vi "Downcast Object.vi"(8 "error in (no error)":errorcluster, 9 "Data Type":u8(ring)=2 items=["DTYPE_BU"=2, "DTYPE_WU"=3, "DTYPE_LU"=4, "DTYPE_QU"=5, "DTYPE_OU"=25, "DTYPE_B"=6, "DTYPE_W"=7, "DTYPE_L"=8, "DTYPE_Q"=9, "DTYPE_O"=26, "DTYPE_FLOAT"=52, "DTYPE_DOUBLE"=53, "DTYPE_T"=14, "DTYPE_IDENT"=191, "DTYPE_NID"=192, "DTYPE_PATH"=193, "DTYPE_PARAM"=194, "DTYPE_SIGNAL"=195, "DTYPE_DIMENSION"=196, "DTYPE_WINDOW"=197, "DTYPE_SLOPE"=198, "DTYPE_FUNCTION"=199, "DTYPE_CONGLOM"=200, "DTYPE_RANGE"=201, "DTYPE_ACTION"=202, "DTYPE_DISPATCH"=203, "DTYPE_PROGRAM"=204, "DTYPE_ROUTINE"=205, "DTYPE_PROCEDURE"=206, "DTYPE_METHOD"=207, "DTYPE_DEPENDENCY"=208, "DTYPE_CONDITION"=209, "DTYPE_EVENT"=210, "DTYPE_WITH_UNITS"=211, "DTYPE_CALL"=212, "DTYPE_WITH_ERROR"=213, "DTYPE_LIST"=214, "DTYPE_TUPLE"=215, "DTYPE_DICTIONARY"=216, "DTYPE_POINTER"=51, "DTYPE_DSC"=24], 10 "Class Type":u8(ring)=2 items=["CLASS_S"=1, "CLASS_D"=2, "CLASS_A"=4, "CLASS_R"=194, "CLASS_APD"=196], 11 "Data in":refnum<class "Data.lvclass">) -> (0 "error out":errorcluster, 3 "Data out":refnum<class "Data.lvclass">)   [LabVIEW 2013, in "MDSplus.lvlib" / "Data.lvclass"]
uses:
  <vilib>/MDSplus/Classes/Data_Class/Data.lvclass
  <vilib>/MDSplus/Classes/Data_Class/Scalar_Class/Float32_Class/Float32.lvclass
  <vilib>/MDSplus/Classes/Data_Class/Scalar_Class/Uint8_Class/Uint8.lvclass
  <vilib>/MDSplus/Classes/Data_Class/Scalar_Class/Uint16_Class/Uint16.lvclass
  <vilib>/MDSplus/Classes/Data_Class/Scalar_Class/Uint32_Class/Uint32.lvclass
  <vilib>/MDSplus/Classes/Data_Class/Scalar_Class/Uint64_Class/Uint64.lvclass
  <vilib>/MDSplus/Classes/Data_Class/Scalar_Class/Int8_Class/Int8.lvclass
  <vilib>/MDSplus/Classes/Data_Class/Scalar_Class/Int16_Class/Int16.lvclass
  <vilib>/MDSplus/Classes/Data_Class/Scalar_Class/Int32_Class/Int32.lvclass
  <vilib>/MDSplus/Classes/Data_Class/Scalar_Class/Int64_Class/Int64.lvclass
  <vilib>/MDSplus/Classes/Data_Class/Scalar_Class/String_Class/String.lvclass
  <vilib>/MDSplus/Classes/Data_Class/Scalar_Class/Float64_Class/Float64.lvclass
  <vilib>/MDSplus/Classes/Data_Class/Array_Class/Uint8Array_Class/Uint8Array.lvclass
  <vilib>/MDSplus/Classes/Data_Class/Array_Class/Uint16Array_Class/Uint16Array.lvclass
  <vilib>/MDSplus/Classes/Data_Class/Array_Class/Uint32Array_Class/Uint32Array.lvclass
  <vilib>/MDSplus/Classes/Data_Class/Array_Class/Uint64Array_Class/Uint64Array.lvclass
  <vilib>/MDSplus/Classes/Data_Class/Array_Class/Int8Array_Class/Int8Array.lvclass
  <vilib>/MDSplus/Classes/Data_Class/Array_Class/Int16Array_Class/Int16Array.lvclass
  <vilib>/MDSplus/Classes/Data_Class/Array_Class/Int32Array_Class/Int32Array.lvclass
  <vilib>/MDSplus/Classes/Data_Class/Array_Class/Int64Array_Class/Int64Array.lvclass
  <vilib>/MDSplus/Classes/Data_Class/Array_Class/StringArray_Class/StringArray.lvclass
  <vilib>/MDSplus/Classes/Data_Class/Array_Class/Float32Array_Class/Float32Array.lvclass
  <vilib>/MDSplus/Classes/Data_Class/Array_Class/Float64Array_Class/Float64Array.lvclass
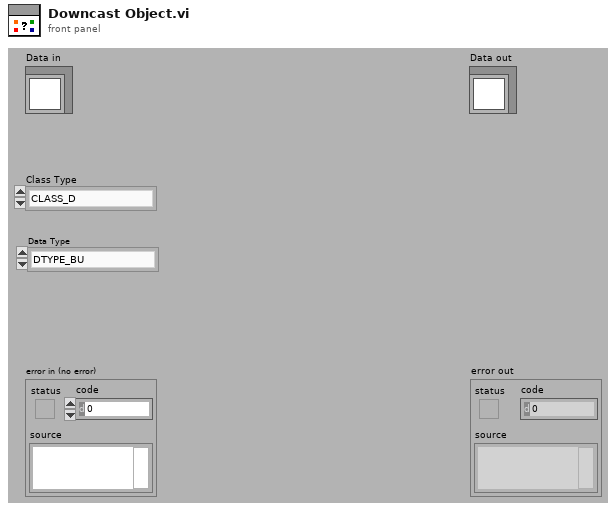
[diagram p1: front panel]
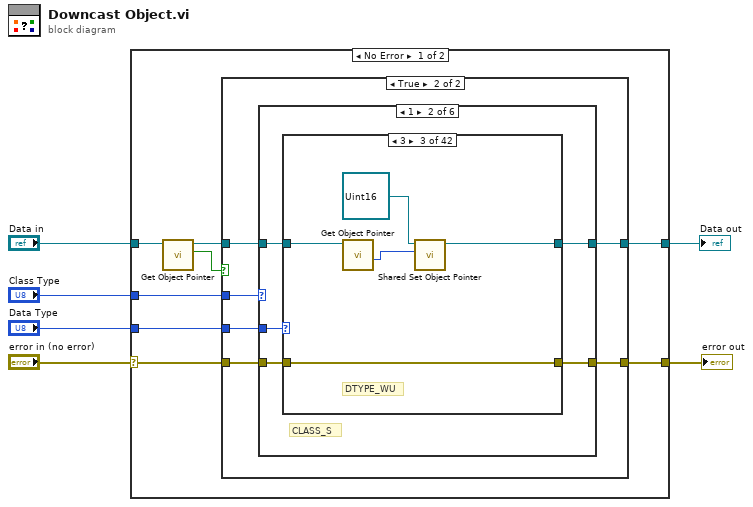
[diagram p0: block diagram]
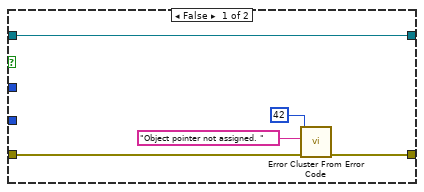
[diagram p2: hidden frame]
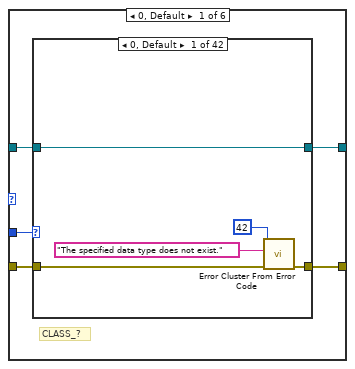
[diagram p3: hidden frame]
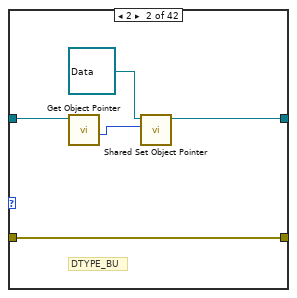
[diagram p4: hidden frame]
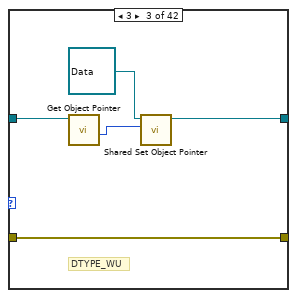
[diagram p5: hidden frame]
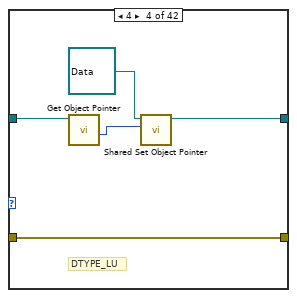
[diagram p6: hidden frame]
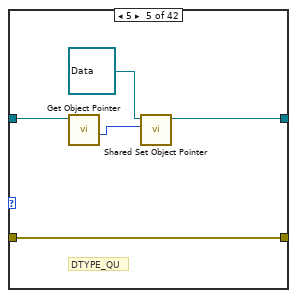
[diagram p7: hidden frame]
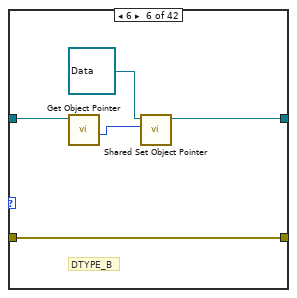
[diagram p8: hidden frame]
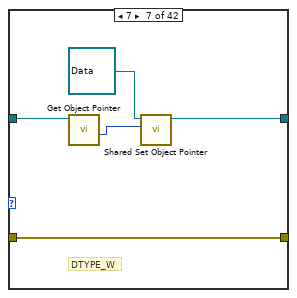
[diagram p9: hidden frame]
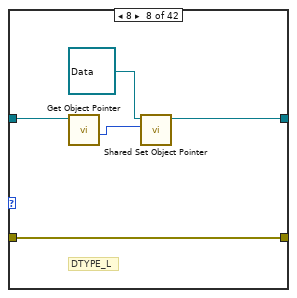
[diagram p10: hidden frame]
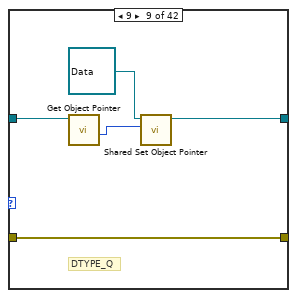
[diagram p11: hidden frame]
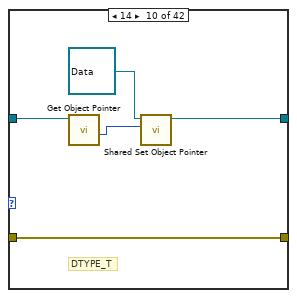
[diagram p12: hidden frame]
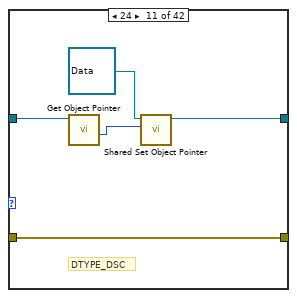
[diagram p13: hidden frame]
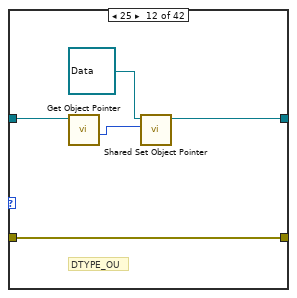
[diagram p14: hidden frame]
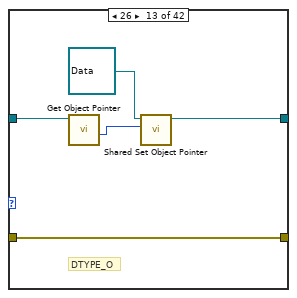
[diagram p15: hidden frame]
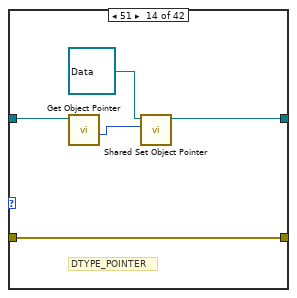
[diagram p16: hidden frame]
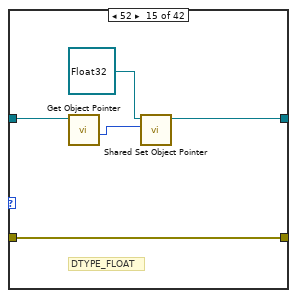
[diagram p17: hidden frame]
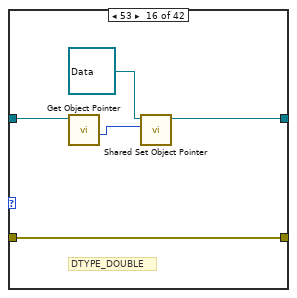
[diagram p18: hidden frame]
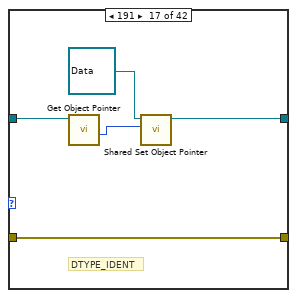
[diagram p19: hidden frame]
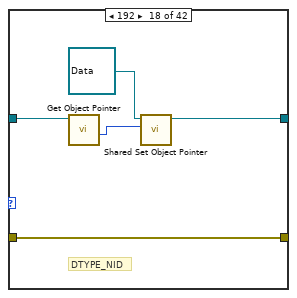
[diagram p20: hidden frame]
diagram:
  n1 = case shown="No Error" "error in (no error)" {
    selector: "error in (no error)" -> [w12 w1317]
    tunnel: [w11 w1317] -> w5
    tunnel: [w10 w1316] -> w3
    tunnel: "Data in" -> [w9 w1316]
    tunnel: "Class Type" -> [w13 _]
    tunnel: "Data Type" -> [w14 _]
    frame No Error {
      n2 = call-dynamic "Get Object Pointer.vi"("Data in"=w9) -> ("Assigned object pointer?"=w7:bool, "Data out"=w8:refnum<class "Data.lvclass">)  [unwired: 8 in, 1 out]
      n3 = case shown="True" w7 {
        tunnel: w14 -> [_ w25]
        tunnel: w13 -> [_ w24]
        tunnel: w12 -> [w17 w23]
        tunnel: [w16 w22] -> w11
        tunnel: [w15 w21] -> w10
        tunnel: w8 -> [w15 w20]
        frame False {
          n4 = call <vilib>:"Error Cluster From Error Code.vi"("error in (no error)"=w17, "error message (\"\")"="Object pointer not assigned. " ("error message (\"\")"), "error code (0)"=42) -> ("error out"=w16:errorcluster)  [unwired: 6 in]
        }
        frame True {
          n5 = case shown="1" w24 {
            tunnel: w20 -> [w27 w242 w457 w672 w887 w1102]
            tunnel: w25 -> [w30 w245 w460 w675 w890 w1105]
            tunnel: w23 -> [w29 w244 w459 w674 w889 w1104]
            tunnel: [w28 w243 w458 w673 w888 w1103] -> w22
            tunnel: [w26 w241 w456 w671 w886 w1101] -> w21
            frame 0, Default {
              # "CLASS_?"
              n6 = case shown="0, Default" w30 {
                tunnel: w29 -> [w35 w37 w42 w47 w52 w57 w62 w67 w72 w77 w82 w87 w92 w97 w102 w107 w112 w117 w122 w127 w132 w137 w142 w147 w152 w157 w162 w167 w172 w177 w182 w187 w192 w197 w202 w207 w212 w217 w222 w227 w232 w237]
                tunnel: [w33 w37 w42 w47 w52 w57 w62 w67 w72 w77 w82 w87 w92 w97 w102 w107 w112 w117 w122 w127 w132 w137 w142 w147 w152 w157 w162 w167 w172 w177 w182 w187 w192 w197 w202 w207 w212 w217 w222 w227 w232 w237] -> w28
                tunnel: [w32 w38 w43 w48 w53 w58 w63 w68 w73 w78 w83 w88 w93 w98 w104 w109 w114 w119 w124 w129 w134 w139 w144 w149 w154 w159 w164 w169 w174 w179 w184 w189 w194 w199 w204 w209 w214 w219 w224 w229 w234 w239] -> w26
                tunnel: w27 -> [w32 w40 w44 w49 w54 w59 w64 w69 w74 w79 w84 w89 w94 w99 w105 w110 w115 w120 w125 w130 w135 w140 w145 w150 w155 w160 w165 w170 w175 w180 w185 w190 w195 w200 w205 w210 w215 w220 w225 w230 w235 w240]
                frame 0, Default {
                  n7 = call <vilib>:"Error Cluster From Error Code.vi"("error in (no error)"=w35, "error message (\"\")"="The specified data type does not exist." ("error message (\"\")"), "error code (0)"=42) -> ("error out"=w33:errorcluster)  [unwired: 6 in]
                }
                frame 2 {
                  # "DTYPE_BU"
                  n8 = call-dynamic "Get Object Pointer.vi"("Data in"=w40) -> ("Object Pointer"=w36:i64)  [unwired: 8 in, 2 out]
                  n9 = call <vilib>:"Shared Set Object Pointer.vi"("Object Pointer"=w36, "Data in"=refnum<class "Data.lvclass"> refnum ("Data.lvclass")) -> ("Data out"=w38:refnum<class "Data.lvclass">)  [unwired: 9 in]
                }
                frame 3 {
                  # "DTYPE_WU"
                  n10 = call-dynamic "Get Object Pointer.vi"("Data in"=w44) -> ("Object Pointer"=w41:i64)  [unwired: 8 in, 2 out]
                  n11 = call <vilib>:"Shared Set Object Pointer.vi"("Object Pointer"=w41, "Data in"=refnum<class "Data.lvclass"> refnum ("Data.lvclass")) -> ("Data out"=w43:refnum<class "Data.lvclass">)  [unwired: 9 in]
                }
                frame 4 {
                  # "DTYPE_LU"
                  n12 = call-dynamic "Get Object Pointer.vi"("Data in"=w49) -> ("Object Pointer"=w46:i64)  [unwired: 8 in, 2 out]
                  n13 = call <vilib>:"Shared Set Object Pointer.vi"("Object Pointer"=w46, "Data in"=refnum<class "Data.lvclass"> refnum ("Data.lvclass")) -> ("Data out"=w48:refnum<class "Data.lvclass">)  [unwired: 9 in]
                }
                frame 5 {
                  # "DTYPE_QU"
                  n14 = call-dynamic "Get Object Pointer.vi"("Data in"=w54) -> ("Object Pointer"=w51:i64)  [unwired: 8 in, 2 out]
                  n15 = call <vilib>:"Shared Set Object Pointer.vi"("Object Pointer"=w51, "Data in"=refnum<class "Data.lvclass"> refnum ("Data.lvclass")) -> ("Data out"=w53:refnum<class "Data.lvclass">)  [unwired: 9 in]
                }
                frame 6 {
                  # "DTYPE_B"
                  n16 = call-dynamic "Get Object Pointer.vi"("Data in"=w59) -> ("Object Pointer"=w56:i64)  [unwired: 8 in, 2 out]
                  n17 = call <vilib>:"Shared Set Object Pointer.vi"("Object Pointer"=w56, "Data in"=refnum<class "Data.lvclass"> refnum ("Data.lvclass")) -> ("Data out"=w58:refnum<class "Data.lvclass">)  [unwired: 9 in]
                }
                frame 7 {
                  # "DTYPE_W"
                  n18 = call-dynamic "Get Object Pointer.vi"("Data in"=w64) -> ("Object Pointer"=w61:i64)  [unwired: 8 in, 2 out]
                  n19 = call <vilib>:"Shared Set Object Pointer.vi"("Object Pointer"=w61, "Data in"=refnum<class "Data.lvclass"> refnum ("Data.lvclass")) -> ("Data out"=w63:refnum<class "Data.lvclass">)  [unwired: 9 in]
                }
                frame 8 {
                  # "DTYPE_L"
                  n20 = call-dynamic "Get Object Pointer.vi"("Data in"=w69) -> ("Object Pointer"=w66:i64)  [unwired: 8 in, 2 out]
                  n21 = call <vilib>:"Shared Set Object Pointer.vi"("Object Pointer"=w66, "Data in"=refnum<class "Data.lvclass"> refnum ("Data.lvclass")) -> ("Data out"=w68:refnum<class "Data.lvclass">)  [unwired: 9 in]
                }
                frame 9 {
                  # "DTYPE_Q"
                  n22 = call-dynamic "Get Object Pointer.vi"("Data in"=w74) -> ("Object Pointer"=w71:i64)  [unwired: 8 in, 2 out]
                  n23 = call <vilib>:"Shared Set Object Pointer.vi"("Object Pointer"=w71, "Data in"=refnum<class "Data.lvclass"> refnum ("Data.lvclass")) -> ("Data out"=w73:refnum<class "Data.lvclass">)  [unwired: 9 in]
                }
                frame 14 {
                  # "DTYPE_T"
                  n24 = call-dynamic "Get Object Pointer.vi"("Data in"=w79) -> ("Object Pointer"=w76:i64)  [unwired: 8 in, 2 out]
                  n25 = call <vilib>:"Shared Set Object Pointer.vi"("Object Pointer"=w76, "Data in"=refnum<class "Data.lvclass"> refnum ("Data.lvclass")) -> ("Data out"=w78:refnum<class "Data.lvclass">)  [unwired: 9 in]
                }
                frame 24 {
                  # "DTYPE_DSC"
                  n26 = call-dynamic "Get Object Pointer.vi"("Data in"=w84) -> ("Object Pointer"=w81:i64)  [unwired: 8 in, 2 out]
                  n27 = call <vilib>:"Shared Set Object Pointer.vi"("Object Pointer"=w81, "Data in"=refnum<class "Data.lvclass"> refnum ("Data.lvclass")) -> ("Data out"=w83:refnum<class "Data.lvclass">)  [unwired: 9 in]
                }
                frame 25 {
                  # "DTYPE_OU"
                  n28 = call-dynamic "Get Object Pointer.vi"("Data in"=w89) -> ("Object Pointer"=w86:i64)  [unwired: 8 in, 2 out]
                  n29 = call <vilib>:"Shared Set Object Pointer.vi"("Object Pointer"=w86, "Data in"=refnum<class "Data.lvclass"> refnum ("Data.lvclass")) -> ("Data out"=w88:refnum<class "Data.lvclass">)  [unwired: 9 in]
                }
                frame 26 {
                  # "DTYPE_O"
                  n30 = call-dynamic "Get Object Pointer.vi"("Data in"=w94) -> ("Object Pointer"=w91:i64)  [unwired: 8 in, 2 out]
                  n31 = call <vilib>:"Shared Set Object Pointer.vi"("Object Pointer"=w91, "Data in"=refnum<class "Data.lvclass"> refnum ("Data.lvclass")) -> ("Data out"=w93:refnum<class "Data.lvclass">)  [unwired: 9 in]
                }
                frame 51 {
                  # "DTYPE_POINTER"
                  n32 = call-dynamic "Get Object Pointer.vi"("Data in"=w99) -> ("Object Pointer"=w96:i64)  [unwired: 8 in, 2 out]
                  n33 = call <vilib>:"Shared Set Object Pointer.vi"("Object Pointer"=w96, "Data in"=refnum<class "Data.lvclass"> refnum ("Data.lvclass")) -> ("Data out"=w98:refnum<class "Data.lvclass">)  [unwired: 9 in]
                }
                frame 52 {
                  # "DTYPE_FLOAT"
                  n34 = call-dynamic "Get Object Pointer.vi"("Data in"=w105) -> ("Object Pointer"=w101:i64)  [unwired: 8 in, 2 out]
                  n35 = call <vilib>:"Shared Set Object Pointer.vi"("Object Pointer"=w101, "Data in"=refnum<class "Float32.lvclass"> refnum ("Float32.lvclass")) -> ("Data out"=w104:refnum<class "Float32.lvclass">)  [unwired: 9 in]
                }
                frame 53 {
                  # "DTYPE_DOUBLE"
                  n36 = call-dynamic "Get Object Pointer.vi"("Data in"=w110) -> ("Object Pointer"=w106:i64)  [unwired: 8 in, 2 out]
                  n37 = call <vilib>:"Shared Set Object Pointer.vi"("Object Pointer"=w106, "Data in"=refnum<class "Data.lvclass"> refnum ("Data.lvclass")) -> ("Data out"=w109:refnum<class "Data.lvclass">)  [unwired: 9 in]
                }
                frame 191 {
                  # "DTYPE_IDENT"
                  n38 = call-dynamic "Get Object Pointer.vi"("Data in"=w115) -> ("Object Pointer"=w111:i64)  [unwired: 8 in, 2 out]
                  n39 = call <vilib>:"Shared Set Object Pointer.vi"("Object Pointer"=w111, "Data in"=refnum<class "Data.lvclass"> refnum ("Data.lvclass")) -> ("Data out"=w114:refnum<class "Data.lvclass">)  [unwired: 9 in]
                }
                frame 192 {
                  # "DTYPE_NID"
                  n40 = call-dynamic "Get Object Pointer.vi"("Data in"=w120) -> ("Object Pointer"=w116:i64)  [unwired: 8 in, 2 out]
                  n41 = call <vilib>:"Shared Set Object Pointer.vi"("Object Pointer"=w116, "Data in"=refnum<class "Data.lvclass"> refnum ("Data.lvclass")) -> ("Data out"=w119:refnum<class "Data.lvclass">)  [unwired: 9 in]
                }
                frame 193 {
                  # "DTYPE_PATH"
                  n42 = call-dynamic "Get Object Pointer.vi"("Data in"=w125) -> ("Object Pointer"=w121:i64)  [unwired: 8 in, 2 out]
                  n43 = call <vilib>:"Shared Set Object Pointer.vi"("Object Pointer"=w121, "Data in"=refnum<class "Data.lvclass"> refnum ("Data.lvclass")) -> ("Data out"=w124:refnum<class "Data.lvclass">)  [unwired: 9 in]
                }
                frame 194 {
                  # "DTYPE_PARAM"
                  n44 = call-dynamic "Get Object Pointer.vi"("Data in"=w130) -> ("Object Pointer"=w126:i64)  [unwired: 8 in, 2 out]
                  n45 = call <vilib>:"Shared Set Object Pointer.vi"("Object Pointer"=w126, "Data in"=refnum<class "Data.lvclass"> refnum ("Data.lvclass")) -> ("Data out"=w129:refnum<class "Data.lvclass">)  [unwired: 9 in]
                }
                frame 195 {
                  # "DTYPE_SIGNAL"
                  n46 = call-dynamic "Get Object Pointer.vi"("Data in"=w135) -> ("Object Pointer"=w131:i64)  [unwired: 8 in, 2 out]
                  n47 = call <vilib>:"Shared Set Object Pointer.vi"("Object Pointer"=w131, "Data in"=refnum<class "Data.lvclass"> refnum ("Data.lvclass")) -> ("Data out"=w134:refnum<class "Data.lvclass">)  [unwired: 9 in]
                }
                frame 196 {
                  # "DTYPE_DIMENSION"
                  n48 = call-dynamic "Get Object Pointer.vi"("Data in"=w140) -> ("Object Pointer"=w136:i64)  [unwired: 8 in, 2 out]
                  n49 = call <vilib>:"Shared Set Object Pointer.vi"("Object Pointer"=w136, "Data in"=refnum<class "Data.lvclass"> refnum ("Data.lvclass")) -> ("Data out"=w139:refnum<class "Data.lvclass">)  [unwired: 9 in]
                }
                frame 197 {
                  # "DTYPE_WINDOW"
                  n50 = call-dynamic "Get Object Pointer.vi"("Data in"=w145) -> ("Object Pointer"=w141:i64)  [unwired: 8 in, 2 out]
                  n51 = call <vilib>:"Shared Set Object Pointer.vi"("Object Pointer"=w141, "Data in"=refnum<class "Data.lvclass"> refnum ("Data.lvclass")) -> ("Data out"=w144:refnum<class "Data.lvclass">)  [unwired: 9 in]
                }
                frame 198 {
                  # "DTYPE_SLOPE"
                  n52 = call-dynamic "Get Object Pointer.vi"("Data in"=w150) -> ("Object Pointer"=w146:i64)  [unwired: 8 in, 2 out]
                  n53 = call <vilib>:"Shared Set Object Pointer.vi"("Object Pointer"=w146, "Data in"=refnum<class "Data.lvclass"> refnum ("Data.lvclass")) -> ("Data out"=w149:refnum<class "Data.lvclass">)  [unwired: 9 in]
                }
                frame 199 {
                  # "DTYPE_FUNCTION"
                  n54 = call-dynamic "Get Object Pointer.vi"("Data in"=w155) -> ("Object Pointer"=w151:i64)  [unwired: 8 in, 2 out]
                  n55 = call <vilib>:"Shared Set Object Pointer.vi"("Object Pointer"=w151, "Data in"=refnum<class "Data.lvclass"> refnum ("Data.lvclass")) -> ("Data out"=w154:refnum<class "Data.lvclass">)  [unwired: 9 in]
                }
                frame 200 {
                  # "DTYPE_CONGLOM"
                  n56 = call-dynamic "Get Object Pointer.vi"("Data in"=w160) -> ("Object Pointer"=w156:i64)  [unwired: 8 in, 2 out]
                  n57 = call <vilib>:"Shared Set Object Pointer.vi"("Object Pointer"=w156, "Data in"=refnum<class "Data.lvclass"> refnum ("Data.lvclass")) -> ("Data out"=w159:refnum<class "Data.lvclass">)  [unwired: 9 in]
                }
                frame 201 {
                  # "DTYPE_RANGE"
                  n58 = call-dynamic "Get Object Pointer.vi"("Data in"=w165) -> ("Object Pointer"=w161:i64)  [unwired: 8 in, 2 out]
                  n59 = call <vilib>:"Shared Set Object Pointer.vi"("Object Pointer"=w161, "Data in"=refnum<class "Data.lvclass"> refnum ("Data.lvclass")) -> ("Data out"=w164:refnum<class "Data.lvclass">)  [unwired: 9 in]
                }
                frame 202 {
                  # "DTYPE_ACTION"
                  n60 = call-dynamic "Get Object Pointer.vi"("Data in"=w170) -> ("Object Pointer"=w166:i64)  [unwired: 8 in, 2 out]
                  n61 = call <vilib>:"Shared Set Object Pointer.vi"("Object Pointer"=w166, "Data in"=refnum<class "Data.lvclass"> refnum ("Data.lvclass")) -> ("Data out"=w169:refnum<class "Data.lvclass">)  [unwired: 9 in]
                }
                frame 203 {
                  # "DTYPE_DISPATCH"
                  n62 = call-dynamic "Get Object Pointer.vi"("Data in"=w175) -> ("Object Pointer"=w171:i64)  [unwired: 8 in, 2 out]
                  n63 = call <vilib>:"Shared Set Object Pointer.vi"("Object Pointer"=w171, "Data in"=refnum<class "Data.lvclass"> refnum ("Data.lvclass")) -> ("Data out"=w174:refnum<class "Data.lvclass">)  [unwired: 9 in]
                }
                frame 204 {
                  # "DTYPE_PROGRAM"
                  n64 = call-dynamic "Get Object Pointer.vi"("Data in"=w180) -> ("Object Pointer"=w176:i64)  [unwired: 8 in, 2 out]
                  n65 = call <vilib>:"Shared Set Object Pointer.vi"("Object Pointer"=w176, "Data in"=refnum<class "Data.lvclass"> refnum ("Data.lvclass")) -> ("Data out"=w179:refnum<class "Data.lvclass">)  [unwired: 9 in]
                }
                frame 205 {
                  # "DTYPE_ROUTINE"
                  n66 = call-dynamic "Get Object Pointer.vi"("Data in"=w185) -> ("Object Pointer"=w181:i64)  [unwired: 8 in, 2 out]
                  n67 = call <vilib>:"Shared Set Object Pointer.vi"("Object Pointer"=w181, "Data in"=refnum<class "Data.lvclass"> refnum ("Data.lvclass")) -> ("Data out"=w184:refnum<class "Data.lvclass">)  [unwired: 9 in]
                }
                frame 206 {
                  # "DTYPE_PROCEDURE"
                  n68 = call-dynamic "Get Object Pointer.vi"("Data in"=w190) -> ("Object Pointer"=w186:i64)  [unwired: 8 in, 2 out]
                  n69 = call <vilib>:"Shared Set Object Pointer.vi"("Object Pointer"=w186, "Data in"=refnum<class "Data.lvclass"> refnum ("Data.lvclass")) -> ("Data out"=w189:refnum<class "Data.lvclass">)  [unwired: 9 in]
                }
                frame 207 {
                  # "DTYPE_METHOD"
                  n70 = call-dynamic "Get Object Pointer.vi"("Data in"=w195) -> ("Object Pointer"=w191:i64)  [unwired: 8 in, 2 out]
                  n71 = call <vilib>:"Shared Set Object Pointer.vi"("Object Pointer"=w191, "Data in"=refnum<class "Data.lvclass"> refnum ("Data.lvclass")) -> ("Data out"=w194:refnum<class "Data.lvclass">)  [unwired: 9 in]
                }
                frame 208 {
                  # "DTYPE_DEPENDENCY"
                  n72 = call-dynamic "Get Object Pointer.vi"("Data in"=w200) -> ("Object Pointer"=w196:i64)  [unwired: 8 in, 2 out]
                  n73 = call <vilib>:"Shared Set Object Pointer.vi"("Object Pointer"=w196, "Data in"=refnum<class "Data.lvclass"> refnum ("Data.lvclass")) -> ("Data out"=w199:refnum<class "Data.lvclass">)  [unwired: 9 in]
                }
                frame 209 {
                  # "DTYPE_CONDITION"
                  n74 = call-dynamic "Get Object Pointer.vi"("Data in"=w205) -> ("Object Pointer"=w201:i64)  [unwired: 8 in, 2 out]
                  n75 = call <vilib>:"Shared Set Object Pointer.vi"("Object Pointer"=w201, "Data in"=refnum<class "Data.lvclass"> refnum ("Data.lvclass")) -> ("Data out"=w204:refnum<class "Data.lvclass">)  [unwired: 9 in]
                }
                frame 210 {
                  # "DTYPE_EVENT"
                  n76 = call-dynamic "Get Object Pointer.vi"("Data in"=w210) -> ("Object Pointer"=w206:i64)  [unwired: 8 in, 2 out]
                  n77 = call <vilib>:"Shared Set Object Pointer.vi"("Object Pointer"=w206, "Data in"=refnum<class "Data.lvclass"> refnum ("Data.lvclass")) -> ("Data out"=w209:refnum<class "Data.lvclass">)  [unwired: 9 in]
                }
                frame 211 {
                  # "DTYPE_WITH_UNITS"
                  n78 = call-dynamic "Get Object Pointer.vi"("Data in"=w215) -> ("Object Pointer"=w211:i64)  [unwired: 8 in, 2 out]
                  n79 = call <vilib>:"Shared Set Object Pointer.vi"("Object Pointer"=w211, "Data in"=refnum<class "Data.lvclass"> refnum ("Data.lvclass")) -> ("Data out"=w214:refnum<class "Data.lvclass">)  [unwired: 9 in]
                }
                frame 212 {
                  # "DTYPE_CALL"
                  n80 = call-dynamic "Get Object Pointer.vi"("Data in"=w220) -> ("Object Pointer"=w216:i64)  [unwired: 8 in, 2 out]
                  n81 = call <vilib>:"Shared Set Object Pointer.vi"("Object Pointer"=w216, "Data in"=refnum<class "Data.lvclass"> refnum ("Data.lvclass")) -> ("Data out"=w219:refnum<class "Data.lvclass">)  [unwired: 9 in]
                }
                frame 213 {
                  # "DTYPE_WITH_ERROR"
                  n82 = call-dynamic "Get Object Pointer.vi"("Data in"=w225) -> ("Object Pointer"=w221:i64)  [unwired: 8 in, 2 out]
                  n83 = call <vilib>:"Shared Set Object Pointer.vi"("Object Pointer"=w221, "Data in"=refnum<class "Data.lvclass"> refnum ("Data.lvclass")) -> ("Data out"=w224:refnum<class "Data.lvclass">)  [unwired: 9 in]
                }
                frame 214 {
                  # "DTYPE_LIST"
                  n84 = call-dynamic "Get Object Pointer.vi"("Data in"=w230) -> ("Object Pointer"=w226:i64)  [unwired: 8 in, 2 out]
                  n85 = call <vilib>:"Shared Set Object Pointer.vi"("Object Pointer"=w226, "Data in"=refnum<class "Data.lvclass"> refnum ("Data.lvclass")) -> ("Data out"=w229:refnum<class "Data.lvclass">)  [unwired: 9 in]
                }
                frame 215 {
                  # "DTYPE_TUPLE"
                  n86 = call-dynamic "Get Object Pointer.vi"("Data in"=w235) -> ("Object Pointer"=w231:i64)  [unwired: 8 in, 2 out]
                  n87 = call <vilib>:"Shared Set Object Pointer.vi"("Object Pointer"=w231, "Data in"=refnum<class "Data.lvclass"> refnum ("Data.lvclass")) -> ("Data out"=w234:refnum<class "Data.lvclass">)  [unwired: 9 in]
                }
                frame 216 {
                  # "DTYPE_DICTIONARY"
                  n88 = call-dynamic "Get Object Pointer.vi"("Data in"=w240) -> ("Object Pointer"=w236:i64)  [unwired: 8 in, 2 out]
                  n89 = call <vilib>:"Shared Set Object Pointer.vi"("Object Pointer"=w236, "Data in"=refnum<class "Data.lvclass"> refnum ("Data.lvclass")) -> ("Data out"=w239:refnum<class "Data.lvclass">)  [unwired: 9 in]
                }
              }
            }
            frame 1 {
              # "CLASS_S"
              n90 = case shown="3" w245 {
                tunnel: w244 -> [w250 w252 w257 w262 w267 w272 w277 w282 w287 w292 w297 w302 w307 w312 w317 w322 w327 w332 w337 w342 w347 w352 w357 w362 w367 w372 w377 w382 w387 w392 w397 w402 w407 w412 w417 w422 w427 w432 w437 w442 w447 w452]
                tunnel: [w248 w252 w257 w262 w267 w272 w277 w282 w287 w292 w297 w302 w307 w312 w317 w322 w327 w332 w337 w342 w347 w352 w357 w362 w367 w372 w377 w382 w387 w392 w397 w402 w407 w412 w417 w422 w427 w432 w437 w442 w447 w452] -> w243
                tunnel: [w247 w253 w258 w263 w268 w273 w278 w283 w288 w293 w298 w303 w308 w313 w319 w324 w329 w334 w339 w344 w349 w354 w359 w364 w369 w374 w379 w384 w389 w394 w399 w404 w409 w414 w419 w424 w429 w434 w439 w444 w449 w454] -> w241
                tunnel: w242 -> [w247 w255 w259 w264 w269 w274 w279 w284 w289 w294 w299 w304 w309 w314 w320 w325 w330 w335 w340 w345 w350 w355 w360 w365 w370 w375 w380 w385 w390 w395 w400 w405 w410 w415 w420 w425 w430 w435 w440 w445 w450 w455]
                frame 0, Default {
                  n91 = call <vilib>:"Error Cluster From Error Code.vi"("error in (no error)"=w250, "error message (\"\")"="The specified data type does not exist." ("error message (\"\")"), "error code (0)"=42) -> ("error out"=w248:errorcluster)  [unwired: 6 in]
                }
                frame 2 {
                  # "DTYPE_BU"
                  n92 = call-dynamic "Get Object Pointer.vi"("Data in"=w255) -> ("Object Pointer"=w251:i64)  [unwired: 8 in, 2 out]
                  n93 = call <vilib>:"Shared Set Object Pointer.vi"("Object Pointer"=w251, "Data in"=refnum<class "Uint8.lvclass"> refnum ("Data.lvclass")) -> ("Data out"=w253:refnum<class "Uint8.lvclass">)  [unwired: 9 in]
                }
                frame 3 {
                  # "DTYPE_WU"
                  n94 = call-dynamic "Get Object Pointer.vi"("Data in"=w259) -> ("Object Pointer"=w256:i64)  [unwired: 8 in, 2 out]
                  n95 = call <vilib>:"Shared Set Object Pointer.vi"("Object Pointer"=w256, "Data in"=refnum<class "Uint16.lvclass"> refnum ("Data.lvclass")) -> ("Data out"=w258:refnum<class "Uint16.lvclass">)  [unwired: 9 in]
                }
                frame 4 {
                  # "DTYPE_LU"
                  n96 = call-dynamic "Get Object Pointer.vi"("Data in"=w264) -> ("Object Pointer"=w261:i64)  [unwired: 8 in, 2 out]
                  n97 = call <vilib>:"Shared Set Object Pointer.vi"("Object Pointer"=w261, "Data in"=refnum<class "Uint32.lvclass"> refnum ("Data.lvclass")) -> ("Data out"=w263:refnum<class "Uint32.lvclass">)  [unwired: 9 in]
                }
                frame 5 {
                  # "DTYPE_QU"
                  n98 = call-dynamic "Get Object Pointer.vi"("Data in"=w269) -> ("Object Pointer"=w266:i64)  [unwired: 8 in, 2 out]
                  n99 = call <vilib>:"Shared Set Object Pointer.vi"("Object Pointer"=w266, "Data in"=refnum<class "Uint64.lvclass"> refnum ("Data.lvclass")) -> ("Data out"=w268:refnum<class "Uint64.lvclass">)  [unwired: 9 in]
                }
                frame 6 {
                  # "DTYPE_B"
                  n100 = call-dynamic "Get Object Pointer.vi"("Data in"=w274) -> ("Object Pointer"=w271:i64)  [unwired: 8 in, 2 out]
                  n101 = call <vilib>:"Shared Set Object Pointer.vi"("Object Pointer"=w271, "Data in"=refnum<class "Int8.lvclass"> refnum ("Data.lvclass")) -> ("Data out"=w273:refnum<class "Int8.lvclass">)  [unwired: 9 in]
                }
                frame 7 {
                  # "DTYPE_W"
                  n102 = call-dynamic "Get Object Pointer.vi"("Data in"=w279) -> ("Object Pointer"=w276:i64)  [unwired: 8 in, 2 out]
                  n103 = call <vilib>:"Shared Set Object Pointer.vi"("Object Pointer"=w276, "Data in"=refnum<class "Int16.lvclass"> refnum ("Data.lvclass")) -> ("Data out"=w278:refnum<class "Int16.lvclass">)  [unwired: 9 in]
                }
                frame 8 {
                  # "DTYPE_L"
                  n104 = call-dynamic "Get Object Pointer.vi"("Data in"=w284) -> ("Object Pointer"=w281:i64)  [unwired: 8 in, 2 out]
                  n105 = call <vilib>:"Shared Set Object Pointer.vi"("Object Pointer"=w281, "Data in"=refnum<class "Int32.lvclass"> refnum ("Data.lvclass")) -> ("Data out"=w283:refnum<class "Int32.lvclass">)  [unwired: 9 in]
                }
                frame 9 {
                  # "DTYPE_Q"
                  n106 = call-dynamic "Get Object Pointer.vi"("Data in"=w289) -> ("Object Pointer"=w286:i64)  [unwired: 8 in, 2 out]
                  n107 = call <vilib>:"Shared Set Object Pointer.vi"("Object Pointer"=w286, "Data in"=refnum<class "Int64.lvclass"> refnum ("Data.lvclass")) -> ("Data out"=w288:refnum<class "Int64.lvclass">)  [unwired: 9 in]
                }
                frame 14 {
                  # "DTYPE_T"
                  n108 = call-dynamic "Get Object Pointer.vi"("Data in"=w294) -> ("Object Pointer"=w291:i64)  [unwired: 8 in, 2 out]
                  n109 = call <vilib>:"Shared Set Object Pointer.vi"("Object Pointer"=w291, "Data in"=refnum<class "String.lvclass"> refnum ("Data.lvclass")) -> ("Data out"=w293:refnum<class "String.lvclass">)  [unwired: 9 in]
                }
                frame 24 {
                  # "DTYPE_DSC"
                  n110 = call-dynamic "Get Object Pointer.vi"("Data in"=w299) -> ("Object Pointer"=w296:i64)  [unwired: 8 in, 2 out]
                  n111 = call <vilib>:"Shared Set Object Pointer.vi"("Object Pointer"=w296, "Data in"=refnum<class "Data.lvclass"> refnum ("Data.lvclass")) -> ("Data out"=w298:refnum<class "Data.lvclass">)  [unwired: 9 in]
                }
                frame 25 {
                  # "DTYPE_OU"
                  n112 = call-dynamic "Get Object Pointer.vi"("Data in"=w304) -> ("Object Pointer"=w301:i64)  [unwired: 8 in, 2 out]
                  n113 = call <vilib>:"Shared Set Object Pointer.vi"("Object Pointer"=w301, "Data in"=refnum<class "Data.lvclass"> refnum ("Data.lvclass")) -> ("Data out"=w303:refnum<class "Data.lvclass">)  [unwired: 9 in]
                }
                frame 26 {
                  # "DTYPE_O"
                  n114 = call-dynamic "Get Object Pointer.vi"("Data in"=w309) -> ("Object Pointer"=w306:i64)  [unwired: 8 in, 2 out]
                  n115 = call <vilib>:"Shared Set Object Pointer.vi"("Object Pointer"=w306, "Data in"=refnum<class "Data.lvclass"> refnum ("Data.lvclass")) -> ("Data out"=w308:refnum<class "Data.lvclass">)  [unwired: 9 in]
                }
                frame 51 {
                  # "DTYPE_POINTER"
                  n116 = call-dynamic "Get Object Pointer.vi"("Data in"=w314) -> ("Object Pointer"=w311:i64)  [unwired: 8 in, 2 out]
                  n117 = call <vilib>:"Shared Set Object Pointer.vi"("Object Pointer"=w311, "Data in"=refnum<class "Data.lvclass"> refnum ("Data.lvclass")) -> ("Data out"=w313:refnum<class "Data.lvclass">)  [unwired: 9 in]
                }
                frame 52 {
                  # "DTYPE_FLOAT"
                  n118 = call-dynamic "Get Object Pointer.vi"("Data in"=w320) -> ("Object Pointer"=w316:i64)  [unwired: 8 in, 2 out]
                  n119 = call <vilib>:"Shared Set Object Pointer.vi"("Object Pointer"=w316, "Data in"=refnum<class "Float32.lvclass"> refnum ("Float32.lvclass")) -> ("Data out"=w319:refnum<class "Float32.lvclass">)  [unwired: 9 in]
                }
                frame 53 {
                  # "DTYPE_DOUBLE"
                  n120 = call-dynamic "Get Object Pointer.vi"("Data in"=w325) -> ("Object Pointer"=w321:i64)  [unwired: 8 in, 2 out]
                  n121 = call <vilib>:"Shared Set Object Pointer.vi"("Object Pointer"=w321, "Data in"=refnum<class "Float64.lvclass"> refnum ("Data.lvclass")) -> ("Data out"=w324:refnum<class "Float64.lvclass">)  [unwired: 9 in]
                }
                frame 191 {
                  # "DTYPE_IDENT"
                  n122 = call-dynamic "Get Object Pointer.vi"("Data in"=w330) -> ("Object Pointer"=w326:i64)  [unwired: 8 in, 2 out]
                  n123 = call <vilib>:"Shared Set Object Pointer.vi"("Object Pointer"=w326, "Data in"=refnum<class "Data.lvclass"> refnum ("Data.lvclass")) -> ("Data out"=w329:refnum<class "Data.lvclass">)  [unwired: 9 in]
                }
                frame 192 {
                  # "DTYPE_NID"
                  n124 = call-dynamic "Get Object Pointer.vi"("Data in"=w335) -> ("Object Pointer"=w331:i64)  [unwired: 8 in, 2 out]
                  n125 = call <vilib>:"Shared Set Object Pointer.vi"("Object Pointer"=w331, "Data in"=refnum<class "Data.lvclass"> refnum ("Data.lvclass")) -> ("Data out"=w334:refnum<class "Data.lvclass">)  [unwired: 9 in]
                }
                frame 193 {
                  # "DTYPE_PATH"
                  n126 = call-dynamic "Get Object Pointer.vi"("Data in"=w340) -> ("Object Pointer"=w336:i64)  [unwired: 8 in, 2 out]
                  n127 = call <vilib>:"Shared Set Object Pointer.vi"("Object Pointer"=w336, "Data in"=refnum<class "Data.lvclass"> refnum ("Data.lvclass")) -> ("Data out"=w339:refnum<class "Data.lvclass">)  [unwired: 9 in]
                }
                frame 194 {
                  # "DTYPE_PARAM"
                  n128 = call-dynamic "Get Object Pointer.vi"("Data in"=w345) -> ("Object Pointer"=w341:i64)  [unwired: 8 in, 2 out]
                  n129 = call <vilib>:"Shared Set Object Pointer.vi"("Object Pointer"=w341, "Data in"=refnum<class "Data.lvclass"> refnum ("Data.lvclass")) -> ("Data out"=w344:refnum<class "Data.lvclass">)  [unwired: 9 in]
                }
                frame 195 {
                  # "DTYPE_SIGNAL"
                  n130 = call-dynamic "Get Object Pointer.vi"("Data in"=w350) -> ("Object Pointer"=w346:i64)  [unwired: 8 in, 2 out]
                  n131 = call <vilib>:"Shared Set Object Pointer.vi"("Object Pointer"=w346, "Data in"=refnum<class "Data.lvclass"> refnum ("Data.lvclass")) -> ("Data out"=w349:refnum<class "Data.lvclass">)  [unwired: 9 in]
                }
                frame 196 {
                  # "DTYPE_DIMENSION"
                  n132 = call-dynamic "Get Object Pointer.vi"("Data in"=w355) -> ("Object Pointer"=w351:i64)  [unwired: 8 in, 2 out]
                  n133 = call <vilib>:"Shared Set Object Pointer.vi"("Object Pointer"=w351, "Data in"=refnum<class "Data.lvclass"> refnum ("Data.lvclass")) -> ("Data out"=w354:refnum<class "Data.lvclass">)  [unwired: 9 in]
                }
                frame 197 {
                  # "DTYPE_WINDOW"
                  n134 = call-dynamic "Get Object Pointer.vi"("Data in"=w360) -> ("Object Pointer"=w356:i64)  [unwired: 8 in, 2 out]
                  n135 = call <vilib>:"Shared Set Object Pointer.vi"("Object Pointer"=w356, "Data in"=refnum<class "Data.lvclass"> refnum ("Data.lvclass")) -> ("Data out"=w359:refnum<class "Data.lvclass">)  [unwired: 9 in]
                }
                frame 198 {
                  # "DTYPE_SLOPE"
                  n136 = call-dynamic "Get Object Pointer.vi"("Data in"=w365) -> ("Object Pointer"=w361:i64)  [unwired: 8 in, 2 out]
                  n137 = call <vilib>:"Shared Set Object Pointer.vi"("Object Pointer"=w361, "Data in"=refnum<class "Data.lvclass"> refnum ("Data.lvclass")) -> ("Data out"=w364:refnum<class "Data.lvclass">)  [unwired: 9 in]
                }
                frame 199 {
                  # "DTYPE_FUNCTION"
                  n138 = call-dynamic "Get Object Pointer.vi"("Data in"=w370) -> ("Object Pointer"=w366:i64)  [unwired: 8 in, 2 out]
                  n139 = call <vilib>:"Shared Set Object Pointer.vi"("Object Pointer"=w366, "Data in"=refnum<class "Data.lvclass"> refnum ("Data.lvclass")) -> ("Data out"=w369:refnum<class "Data.lvclass">)  [unwired: 9 in]
                }
                frame 200 {
                  # "DTYPE_CONGLOM"
                  n140 = call-dynamic "Get Object Pointer.vi"("Data in"=w375) -> ("Object Pointer"=w371:i64)  [unwired: 8 in, 2 out]
                  n141 = call <vilib>:"Shared Set Object Pointer.vi"("Object Pointer"=w371, "Data in"=refnum<class "Data.lvclass"> refnum ("Data.lvclass")) -> ("Data out"=w374:refnum<class "Data.lvclass">)  [unwired: 9 in]
                }
                frame 201 {
                  # "DTYPE_RANGE"
                  n142 = call-dynamic "Get Object Pointer.vi"("Data in"=w380) -> ("Object Pointer"=w376:i64)  [unwired: 8 in, 2 out]
                  n143 = call <vilib>:"Shared Set Object Pointer.vi"("Object Pointer"=w376, "Data in"=refnum<class "Data.lvclass"> refnum ("Data.lvclass")) -> ("Data out"=w379:refnum<class "Data.lvclass">)  [unwired: 9 in]
                }
                frame 202 {
                  # "DTYPE_ACTION"
                  n144 = call-dynamic "Get Object Pointer.vi"("Data in"=w385) -> ("Object Pointer"=w381:i64)  [unwired: 8 in, 2 out]
                  n145 = call <vilib>:"Shared Set Object Pointer.vi"("Object Pointer"=w381, "Data in"=refnum<class "Data.lvclass"> refnum ("Data.lvclass")) -> ("Data out"=w384:refnum<class "Data.lvclass">)  [unwired: 9 in]
                }
                frame 203 {
                  # "DTYPE_DISPATCH"
                  n146 = call-dynamic "Get Object Pointer.vi"("Data in"=w390) -> ("Object Pointer"=w386:i64)  [unwired: 8 in, 2 out]
                  n147 = call <vilib>:"Shared Set Object Pointer.vi"("Object Pointer"=w386, "Data in"=refnum<class "Data.lvclass"> refnum ("Data.lvclass")) -> ("Data out"=w389:refnum<class "Data.lvclass">)  [unwired: 9 in]
                }
                frame 204 {
                  # "DTYPE_PROGRAM"
                  n148 = call-dynamic "Get Object Pointer.vi"("Data in"=w395) -> ("Object Pointer"=w391:i64)  [unwired: 8 in, 2 out]
                  n149 = call <vilib>:"Shared Set Object Pointer.vi"("Object Pointer"=w391, "Data in"=refnum<class "Data.lvclass"> refnum ("Data.lvclass")) -> ("Data out"=w394:refnum<class "Data.lvclass">)  [unwired: 9 in]
                }
                frame 205 {
                  # "DTYPE_ROUTINE"
                  n150 = call-dynamic "Get Object Pointer.vi"("Data in"=w400) -> ("Object Pointer"=w396:i64)  [unwired: 8 in, 2 out]
                  n151 = call <vilib>:"Shared Set Object Pointer.vi"("Object Pointer"=w396, "Data in"=refnum<class "Data.lvclass"> refnum ("Data.lvclass")) -> ("Data out"=w399:refnum<class "Data.lvclass">)  [unwired: 9 in]
                }
                frame 206 {
                  # "DTYPE_PROCEDURE"
                  n152 = call-dynamic "Get Object Pointer.vi"("Data in"=w405) -> ("Object Pointer"=w401:i64)  [unwired: 8 in, 2 out]
                  n153 = call <vilib>:"Shared Set Object Pointer.vi"("Object Pointer"=w401, "Data in"=refnum<class "Data.lvclass"> refnum ("Data.lvclass")) -> ("Data out"=w404:refnum<class "Data.lvclass">)  [unwired: 9 in]
                }
                frame 207 {
                  # "DTYPE_METHOD"
                  n154 = call-dynamic "Get Object Pointer.vi"("Data in"=w410) -> ("Object Pointer"=w406:i64)  [unwired: 8 in, 2 out]
                  n155 = call <vilib>:"Shared Set Object Pointer.vi"("Object Pointer"=w406, "Data in"=refnum<class "Data.lvclass"> refnum ("Data.lvclass")) -> ("Data out"=w409:refnum<class "Data.lvclass">)  [unwired: 9 in]
                }
                frame 208 {
                  # "DTYPE_DEPENDENCY"
                  n156 = call-dynamic "Get Object Pointer.vi"("Data in"=w415) -> ("Object Pointer"=w411:i64)  [unwired: 8 in, 2 out]
                  n157 = call <vilib>:"Shared Set Object Pointer.vi"("Object Pointer"=w411, "Data in"=refnum<class "Data.lvclass"> refnum ("Data.lvclass")) -> ("Data out"=w414:refnum<class "Data.lvclass">)  [unwired: 9 in]
                }
                frame 209 {
                  # "DTYPE_CONDITION"
                  n158 = call-dynamic "Get Object Pointer.vi"("Data in"=w420) -> ("Object Pointer"=w416:i64)  [unwired: 8 in, 2 out]
                  n159 = call <vilib>:"Shared Set Object Pointer.vi"("Object Pointer"=w416, "Data in"=refnum<class "Data.lvclass"> refnum ("Data.lvclass")) -> ("Data out"=w419:refnum<class "Data.lvclass">)  [unwired: 9 in]
                }
                frame 210 {
                  # "DTYPE_EVENT"
                  n160 = call-dynamic "Get Object Pointer.vi"("Data in"=w425) -> ("Object Pointer"=w421:i64)  [unwired: 8 in, 2 out]
                  n161 = call <vilib>:"Shared Set Object Pointer.vi"("Object Pointer"=w421, "Data in"=refnum<class "Data.lvclass"> refnum ("Data.lvclass")) -> ("Data out"=w424:refnum<class "Data.lvclass">)  [unwired: 9 in]
                }
                frame 211 {
                  # "DTYPE_WITH_UNITS"
                  n162 = call-dynamic "Get Object Pointer.vi"("Data in"=w430) -> ("Object Pointer"=w426:i64)  [unwired: 8 in, 2 out]
                  n163 = call <vilib>:"Shared Set Object Pointer.vi"("Object Pointer"=w426, "Data in"=refnum<class "Data.lvclass"> refnum ("Data.lvclass")) -> ("Data out"=w429:refnum<class "Data.lvclass">)  [unwired: 9 in]
                }
                frame 212 {
                  # "DTYPE_CALL"
                  n164 = call-dynamic "Get Object Pointer.vi"("Data in"=w435) -> ("Object Pointer"=w431:i64)  [unwired: 8 in, 2 out]
                  n165 = call <vilib>:"Shared Set Object Pointer.vi"("Object Pointer"=w431, "Data in"=refnum<class "Data.lvclass"> refnum ("Data.lvclass")) -> ("Data out"=w434:refnum<class "Data.lvclass">)  [unwired: 9 in]
                }
                frame 213 {
                  # "DTYPE_WITH_ERROR"
                  n166 = call-dynamic "Get Object Pointer.vi"("Data in"=w440) -> ("Object Pointer"=w436:i64)  [unwired: 8 in, 2 out]
                  n167 = call <vilib>:"Shared Set Object Pointer.vi"("Object Pointer"=w436, "Data in"=refnum<class "Data.lvclass"> refnum ("Data.lvclass")) -> ("Data out"=w439:refnum<class "Data.lvclass">)  [unwired: 9 in]
                }
                frame 214 {
                  # "DTYPE_LIST"
                  n168 = call-dynamic "Get Object Pointer.vi"("Data in"=w445) -> ("Object Pointer"=w441:i64)  [unwired: 8 in, 2 out]
                  n169 = call <vilib>:"Shared Set Object Pointer.vi"("Object Pointer"=w441, "Data in"=refnum<class "Data.lvclass"> refnum ("Data.lvclass")) -> ("Data out"=w444:refnum<class "Data.lvclass">)  [unwired: 9 in]
                }
                frame 215 {
                  # "DTYPE_TUPLE"
                  n170 = call-dynamic "Get Object Pointer.vi"("Data in"=w450) -> ("Object Pointer"=w446:i64)  [unwired: 8 in, 2 out]
                  n171 = call <vilib>:"Shared Set Object Pointer.vi"("Object Pointer"=w446, "Data in"=refnum<class "Data.lvclass"> refnum ("Data.lvclass")) -> ("Data out"=w449:refnum<class "Data.lvclass">)  [unwired: 9 in]
                }
                frame 216 {
                  # "DTYPE_DICTIONARY"
                  n172 = call-dynamic "Get Object Pointer.vi"("Data in"=w455) -> ("Object Pointer"=w451:i64)  [unwired: 8 in, 2 out]
                  n173 = call <vilib>:"Shared Set Object Pointer.vi"("Object Pointer"=w451, "Data in"=refnum<class "Data.lvclass"> refnum ("Data.lvclass")) -> ("Data out"=w454:refnum<class "Data.lvclass">)  [unwired: 9 in]
                }
              }
            }
            frame 2 {
              # "CLASS_D"
              n174 = case shown="0, Default" w460 {
                tunnel: w459 -> [w465 w467 w472 w477 w482 w487 w492 w497 w502 w507 w512 w517 w522 w527 w532 w537 w542 w547 w552 w557 w562 w567 w572 w577 w582 w587 w592 w597 w602 w607 w612 w617 w622 w627 w632 w637 w642 w647 w652 w657 w662 w667]
                tunnel: [w463 w467 w472 w477 w482 w487 w492 w497 w502 w507 w512 w517 w522 w527 w532 w537 w542 w547 w552 w557 w562 w567 w572 w577 w582 w587 w592 w597 w602 w607 w612 w617 w622 w627 w632 w637 w642 w647 w652 w657 w662 w667] -> w458
                tunnel: [w462 w468 w473 w478 w483 w488 w493 w498 w503 w508 w513 w518 w523 w528 w534 w539 w544 w549 w554 w559 w564 w569 w574 w579 w584 w589 w594 w599 w604 w609 w614 w619 w624 w629 w634 w639 w644 w649 w654 w659 w664 w669] -> w456
                tunnel: w457 -> [w462 w470 w474 w479 w484 w489 w494 w499 w504 w509 w514 w519 w524 w529 w535 w540 w545 w550 w555 w560 w565 w570 w575 w580 w585 w590 w595 w600 w605 w610 w615 w620 w625 w630 w635 w640 w645 w650 w655 w660 w665 w670]
                frame 0, Default {
                  n175 = call <vilib>:"Error Cluster From Error Code.vi"("error in (no error)"=w465, "error message (\"\")"="The specified data type does not exist." ("error message (\"\")"), "error code (0)"=42) -> ("error out"=w463:errorcluster)  [unwired: 6 in]
                }
                frame 2 {
                  # "DTYPE_BU"
                  n176 = call-dynamic "Get Object Pointer.vi"("Data in"=w470) -> ("Object Pointer"=w466:i64)  [unwired: 8 in, 2 out]
                  n177 = call <vilib>:"Shared Set Object Pointer.vi"("Object Pointer"=w466, "Data in"=refnum<class "Data.lvclass"> refnum ("Data.lvclass")) -> ("Data out"=w468:refnum<class "Data.lvclass">)  [unwired: 9 in]
                }
                frame 3 {
                  # "DTYPE_WU"
                  n178 = call-dynamic "Get Object Pointer.vi"("Data in"=w474) -> ("Object Pointer"=w471:i64)  [unwired: 8 in, 2 out]
                  n179 = call <vilib>:"Shared Set Object Pointer.vi"("Object Pointer"=w471, "Data in"=refnum<class "Data.lvclass"> refnum ("Data.lvclass")) -> ("Data out"=w473:refnum<class "Data.lvclass">)  [unwired: 9 in]
                }
                frame 4 {
                  # "DTYPE_LU"
                  n180 = call-dynamic "Get Object Pointer.vi"("Data in"=w479) -> ("Object Pointer"=w476:i64)  [unwired: 8 in, 2 out]
                  n181 = call <vilib>:"Shared Set Object Pointer.vi"("Object Pointer"=w476, "Data in"=refnum<class "Data.lvclass"> refnum ("Data.lvclass")) -> ("Data out"=w478:refnum<class "Data.lvclass">)  [unwired: 9 in]
                }
                frame 5 {
                  # "DTYPE_QU"
                  n182 = call-dynamic "Get Object Pointer.vi"("Data in"=w484) -> ("Object Pointer"=w481:i64)  [unwired: 8 in, 2 out]
                  n183 = call <vilib>:"Shared Set Object Pointer.vi"("Object Pointer"=w481, "Data in"=refnum<class "Data.lvclass"> refnum ("Data.lvclass")) -> ("Data out"=w483:refnum<class "Data.lvclass">)  [unwired: 9 in]
                }
                frame 6 {
                  # "DTYPE_B"
                  n184 = call-dynamic "Get Object Pointer.vi"("Data in"=w489) -> ("Object Pointer"=w486:i64)  [unwired: 8 in, 2 out]
                  n185 = call <vilib>:"Shared Set Object Pointer.vi"("Object Pointer"=w486, "Data in"=refnum<class "Data.lvclass"> refnum ("Data.lvclass")) -> ("Data out"=w488:refnum<class "Data.lvclass">)  [unwired: 9 in]
                }
                frame 7 {
                  # "DTYPE_W"
                  n186 = call-dynamic "Get Object Pointer.vi"("Data in"=w494) -> ("Object Pointer"=w491:i64)  [unwired: 8 in, 2 out]
                  n187 = call <vilib>:"Shared Set Object Pointer.vi"("Object Pointer"=w491, "Data in"=refnum<class "Data.lvclass"> refnum ("Data.lvclass")) -> ("Data out"=w493:refnum<class "Data.lvclass">)  [unwired: 9 in]
                }
                frame 8 {
                  # "DTYPE_L"
                  n188 = call-dynamic "Get Object Pointer.vi"("Data in"=w499) -> ("Object Pointer"=w496:i64)  [unwired: 8 in, 2 out]
                  n189 = call <vilib>:"Shared Set Object Pointer.vi"("Object Pointer"=w496, "Data in"=refnum<class "Data.lvclass"> refnum ("Data.lvclass")) -> ("Data out"=w498:refnum<class "Data.lvclass">)  [unwired: 9 in]
                }
                frame 9 {
                  # "DTYPE_Q"
                  n190 = call-dynamic "Get Object Pointer.vi"("Data in"=w504) -> ("Object Pointer"=w501:i64)  [unwired: 8 in, 2 out]
                  n191 = call <vilib>:"Shared Set Object Pointer.vi"("Object Pointer"=w501, "Data in"=refnum<class "Data.lvclass"> refnum ("Data.lvclass")) -> ("Data out"=w503:refnum<class "Data.lvclass">)  [unwired: 9 in]
                }
                frame 14 {
                  # "DTYPE_T"
                  n192 = call-dynamic "Get Object Pointer.vi"("Data in"=w509) -> ("Object Pointer"=w506:i64)  [unwired: 8 in, 2 out]
                  n193 = call <vilib>:"Shared Set Object Pointer.vi"("Object Pointer"=w506, "Data in"=refnum<class "Data.lvclass"> refnum ("Data.lvclass")) -> ("Data out"=w508:refnum<class "Data.lvclass">)  [unwired: 9 in]
                }
                frame 24 {
                  # "DTYPE_DSC"
                  n194 = call-dynamic "Get Object Pointer.vi"("Data in"=w514) -> ("Object Pointer"=w511:i64)  [unwired: 8 in, 2 out]
                  n195 = call <vilib>:"Shared Set Object Pointer.vi"("Object Pointer"=w511, "Data in"=refnum<class "Data.lvclass"> refnum ("Data.lvclass")) -> ("Data out"=w513:refnum<class "Data.lvclass">)  [unwired: 9 in]
                }
                frame 25 {
                  # "DTYPE_OU"
                  n196 = call-dynamic "Get Object Pointer.vi"("Data in"=w519) -> ("Object Pointer"=w516:i64)  [unwired: 8 in, 2 out]
                  n197 = call <vilib>:"Shared Set Object Pointer.vi"("Object Pointer"=w516, "Data in"=refnum<class "Data.lvclass"> refnum ("Data.lvclass")) -> ("Data out"=w518:refnum<class "Data.lvclass">)  [unwired: 9 in]
                }
                frame 26 {
                  # "DTYPE_O"
                  n198 = call-dynamic "Get Object Pointer.vi"("Data in"=w524) -> ("Object Pointer"=w521:i64)  [unwired: 8 in, 2 out]
                  n199 = call <vilib>:"Shared Set Object Pointer.vi"("Object Pointer"=w521, "Data in"=refnum<class "Data.lvclass"> refnum ("Data.lvclass")) -> ("Data out"=w523:refnum<class "Data.lvclass">)  [unwired: 9 in]
                }
                frame 51 {
                  # "DTYPE_POINTER"
                  n200 = call-dynamic "Get Object Pointer.vi"("Data in"=w529) -> ("Object Pointer"=w526:i64)  [unwired: 8 in, 2 out]
                  n201 = call <vilib>:"Shared Set Object Pointer.vi"("Object Pointer"=w526, "Data in"=refnum<class "Data.lvclass"> refnum ("Data.lvclass")) -> ("Data out"=w528:refnum<class "Data.lvclass">)  [unwired: 9 in]
                }
                frame 52 {
                  # "DTYPE_FLOAT"
                  n202 = call-dynamic "Get Object Pointer.vi"("Data in"=w535) -> ("Object Pointer"=w531:i64)  [unwired: 8 in, 2 out]
                  n203 = call <vilib>:"Shared Set Object Pointer.vi"("Object Pointer"=w531, "Data in"=refnum<class "Data.lvclass"> refnum ("Data.lvclass")) -> ("Data out"=w534:refnum<class "Data.lvclass">)  [unwired: 9 in]
                }
                frame 53 {
                  # "DTYPE_DOUBLE"
                  n204 = call-dynamic "Get Object Pointer.vi"("Data in"=w540) -> ("Object Pointer"=w536:i64)  [unwired: 8 in, 2 out]
                  n205 = call <vilib>:"Shared Set Object Pointer.vi"("Object Pointer"=w536, "Data in"=refnum<class "Data.lvclass"> refnum ("Data.lvclass")) -> ("Data out"=w539:refnum<class "Data.lvclass">)  [unwired: 9 in]
                }
                frame 191 {
                  # "DTYPE_IDENT"
                  n206 = call-dynamic "Get Object Pointer.vi"("Data in"=w545) -> ("Object Pointer"=w541:i64)  [unwired: 8 in, 2 out]
                  n207 = call <vilib>:"Shared Set Object Pointer.vi"("Object Pointer"=w541, "Data in"=refnum<class "Data.lvclass"> refnum ("Data.lvclass")) -> ("Data out"=w544:refnum<class "Data.lvclass">)  [unwired: 9 in]
                }
                frame 192 {
                  # "DTYPE_NID"
                  n208 = call-dynamic "Get Object Pointer.vi"("Data in"=w550) -> ("Object Pointer"=w546:i64)  [unwired: 8 in, 2 out]
                  n209 = call <vilib>:"Shared Set Object Pointer.vi"("Object Pointer"=w546, "Data in"=refnum<class "Data.lvclass"> refnum ("Data.lvclass")) -> ("Data out"=w549:refnum<class "Data.lvclass">)  [unwired: 9 in]
                }
                frame 193 {
                  # "DTYPE_PATH"
                  n210 = call-dynamic "Get Object Pointer.vi"("Data in"=w555) -> ("Object Pointer"=w551:i64)  [unwired: 8 in, 2 out]
                  n211 = call <vilib>:"Shared Set Object Pointer.vi"("Object Pointer"=w551, "Data in"=refnum<class "Data.lvclass"> refnum ("Data.lvclass")) -> ("Data out"=w554:refnum<class "Data.lvclass">)  [unwired: 9 in]
                }
                frame 194 {
                  # "DTYPE_PARAM"
                  n212 = call-dynamic "Get Object Pointer.vi"("Data in"=w560) -> ("Object Pointer"=w556:i64)  [unwired: 8 in, 2 out]
                  n213 = call <vilib>:"Shared Set Object Pointer.vi"("Object Pointer"=w556, "Data in"=refnum<class "Data.lvclass"> refnum ("Data.lvclass")) -> ("Data out"=w559:refnum<class "Data.lvclass">)  [unwired: 9 in]
                }
                frame 195 {
                  # "DTYPE_SIGNAL"
                  n214 = call-dynamic "Get Object Pointer.vi"("Data in"=w565) -> ("Object Pointer"=w561:i64)  [unwired: 8 in, 2 out]
                  n215 = call <vilib>:"Shared Set Object Pointer.vi"("Object Pointer"=w561, "Data in"=refnum<class "Data.lvclass"> refnum ("Data.lvclass")) -> ("Data out"=w564:refnum<class "Data.lvclass">)  [unwired: 9 in]
                }
                frame 196 {
                  # "DTYPE_DIMENSION"
                  n216 = call-dynamic "Get Object Pointer.vi"("Data in"=w570) -> ("Object Pointer"=w566:i64)  [unwired: 8 in, 2 out]
                  n217 = call <vilib>:"Shared Set Object Pointer.vi"("Object Pointer"=w566, "Data in"=refnum<class "Data.lvclass"> refnum ("Data.lvclass")) -> ("Data out"=w569:refnum<class "Data.lvclass">)  [unwired: 9 in]
                }
                frame 197 {
                  # "DTYPE_WINDOW"
                  n218 = call-dynamic "Get Object Pointer.vi"("Data in"=w575) -> ("Object Pointer"=w571:i64)  [unwired: 8 in, 2 out]
                  n219 = call <vilib>:"Shared Set Object Pointer.vi"("Object Pointer"=w571, "Data in"=refnum<class "Data.lvclass"> refnum ("Data.lvclass")) -> ("Data out"=w574:refnum<class "Data.lvclass">)  [unwired: 9 in]
                }
                frame 198 {
                  # "DTYPE_SLOPE"
                  n220 = call-dynamic "Get Object Pointer.vi"("Data in"=w580) -> ("Object Pointer"=w576:i64)  [unwired: 8 in, 2 out]
                  n221 = call <vilib>:"Shared Set Object Pointer.vi"("Object Pointer"=w576, "Data in"=refnum<class "Data.lvclass"> refnum ("Data.lvclass")) -> ("Data out"=w579:refnum<class "Data.lvclass">)  [unwired: 9 in]
                }
                frame 199 {
                  # "DTYPE_FUNCTION"
                  n222 = call-dynamic "Get Object Pointer.vi"("Data in"=w585) -> ("Object Pointer"=w581:i64)  [unwired: 8 in, 2 out]
                  n223 = call <vilib>:"Shared Set Object Pointer.vi"("Object Pointer"=w581, "Data in"=refnum<class "Data.lvclass"> refnum ("Data.lvclass")) -> ("Data out"=w584:refnum<class "Data.lvclass">)  [unwired: 9 in]
                }
                frame 200 {
                  # "DTYPE_CONGLOM"
                  n224 = call-dynamic "Get Object Pointer.vi"("Data in"=w590) -> ("Object Pointer"=w586:i64)  [unwired: 8 in, 2 out]
                  n225 = call <vilib>:"Shared Set Object Pointer.vi"("Object Pointer"=w586, "Data in"=refnum<class "Data.lvclass"> refnum ("Data.lvclass")) -> ("Data out"=w589:refnum<class "Data.lvclass">)  [unwired: 9 in]
                }
                frame 201 {
                  # "DTYPE_RANGE"
                  n226 = call-dynamic "Get Object Pointer.vi"("Data in"=w595) -> ("Object Pointer"=w591:i64)  [unwired: 8 in, 2 out]
                  n227 = call <vilib>:"Shared Set Object Pointer.vi"("Object Pointer"=w591, "Data in"=refnum<class "Data.lvclass"> refnum ("Data.lvclass")) -> ("Data out"=w594:refnum<class "Data.lvclass">)  [unwired: 9 in]
                }
                frame 202 {
                  # "DTYPE_ACTION"
                  n228 = call-dynamic "Get Object Pointer.vi"("Data in"=w600) -> ("Object Pointer"=w596:i64)  [unwired: 8 in, 2 out]
                  n229 = call <vilib>:"Shared Set Object Pointer.vi"("Object Pointer"=w596, "Data in"=refnum<class "Data.lvclass"> refnum ("Data.lvclass")) -> ("Data out"=w599:refnum<class "Data.lvclass">)  [unwired: 9 in]
                }
                frame 203 {
                  # "DTYPE_DISPATCH"
                  n230 = call-dynamic "Get Object Pointer.vi"("Data in"=w605) -> ("Object Pointer"=w601:i64)  [unwired: 8 in, 2 out]
                  n231 = call <vilib>:"Shared Set Object Pointer.vi"("Object Pointer"=w601, "Data in"=refnum<class "Data.lvclass"> refnum ("Data.lvclass")) -> ("Data out"=w604:refnum<class "Data.lvclass">)  [unwired: 9 in]
                }
                frame 204 {
                  # "DTYPE_PROGRAM"
                  n232 = call-dynamic "Get Object Pointer.vi"("Data in"=w610) -> ("Object Pointer"=w606:i64)  [unwired: 8 in, 2 out]
                  n233 = call <vilib>:"Shared Set Object Pointer.vi"("Object Pointer"=w606, "Data in"=refnum<class "Data.lvclass"> refnum ("Data.lvclass")) -> ("Data out"=w609:refnum<class "Data.lvclass">)  [unwired: 9 in]
                }
                frame 205 {
                  # "DTYPE_ROUTINE"
                  n234 = call-dynamic "Get Object Pointer.vi"("Data in"=w615) -> ("Object Pointer"=w611:i64)  [unwired: 8 in, 2 out]
                  n235 = call <vilib>:"Shared Set Object Pointer.vi"("Object Pointer"=w611, "Data in"=refnum<class "Data.lvclass"> refnum ("Data.lvclass")) -> ("Data out"=w614:refnum<class "Data.lvclass">)  [unwired: 9 in]
                }
                frame 206 {
                  # "DTYPE_PROCEDURE"
                  n236 = call-dynamic "Get Object Pointer.vi"("Data in"=w620) -> ("Object Pointer"=w616:i64)  [unwired: 8 in, 2 out]
                  n237 = call <vilib>:"Shared Set Object Pointer.vi"("Object Pointer"=w616, "Data in"=refnum<class "Data.lvclass"> refnum ("Data.lvclass")) -> ("Data out"=w619:refnum<class "Data.lvclass">)  [unwired: 9 in]
                }
                frame 207 {
                  # "DTYPE_METHOD"
                  n238 = call-dynamic "Get Object Pointer.vi"("Data in"=w625) -> ("Object Pointer"=w621:i64)  [unwired: 8 in, 2 out]
                  n239 = call <vilib>:"Shared Set Object Pointer.vi"("Object Pointer"=w621, "Data in"=refnum<class "Data.lvclass"> refnum ("Data.lvclass")) -> ("Data out"=w624:refnum<class "Data.lvclass">)  [unwired: 9 in]
                }
                frame 208 {
                  # "DTYPE_DEPENDENCY"
                  n240 = call-dynamic "Get Object Pointer.vi"("Data in"=w630) -> ("Object Pointer"=w626:i64)  [unwired: 8 in, 2 out]
                  n241 = call <vilib>:"Shared Set Object Pointer.vi"("Object Pointer"=w626, "Data in"=refnum<class "Data.lvclass"> refnum ("Data.lvclass")) -> ("Data out"=w629:refnum<class "Data.lvclass">)  [unwired: 9 in]
                }
                frame 209 {
                  # "DTYPE_CONDITION"
                  n242 = call-dynamic "Get Object Pointer.vi"("Data in"=w635) -> ("Object Pointer"=w631:i64)  [unwired: 8 in, 2 out]
                  n243 = call <vilib>:"Shared Set Object Pointer.vi"("Object Pointer"=w631, "Data in"=refnum<class "Data.lvclass"> refnum ("Data.lvclass")) -> ("Data out"=w634:refnum<class "Data.lvclass">)  [unwired: 9 in]
                }
                frame 210 {
                  # "DTYPE_EVENT"
                  n244 = call-dynamic "Get Object Pointer.vi"("Data in"=w640) -> ("Object Pointer"=w636:i64)  [unwired: 8 in, 2 out]
                  n245 = call <vilib>:"Shared Set Object Pointer.vi"("Object Pointer"=w636, "Data in"=refnum<class "Data.lvclass"> refnum ("Data.lvclass")) -> ("Data out"=w639:refnum<class "Data.lvclass">)  [unwired: 9 in]
                }
                frame 211 {
                  # "DTYPE_WITH_UNITS"
                  n246 = call-dynamic "Get Object Pointer.vi"("Data in"=w645) -> ("Object Pointer"=w641:i64)  [unwired: 8 in, 2 out]
                  n247 = call <vilib>:"Shared Set Object Pointer.vi"("Object Pointer"=w641, "Data in"=refnum<class "Data.lvclass"> refnum ("Data.lvclass")) -> ("Data out"=w644:refnum<class "Data.lvclass">)  [unwired: 9 in]
                }
                frame 212 {
                  # "DTYPE_CALL"
                  n248 = call-dynamic "Get Object Pointer.vi"("Data in"=w650) -> ("Object Pointer"=w646:i64)  [unwired: 8 in, 2 out]
                  n249 = call <vilib>:"Shared Set Object Pointer.vi"("Object Pointer"=w646, "Data in"=refnum<class "Data.lvclass"> refnum ("Data.lvclass")) -> ("Data out"=w649:refnum<class "Data.lvclass">)  [unwired: 9 in]
                }
                frame 213 {
                  # "DTYPE_WITH_ERROR"
                  n250 = call-dynamic "Get Object Pointer.vi"("Data in"=w655) -> ("Object Pointer"=w651:i64)  [unwired: 8 in, 2 out]
                  n251 = call <vilib>:"Shared Set Object Pointer.vi"("Object Pointer"=w651, "Data in"=refnum<class "Data.lvclass"> refnum ("Data.lvclass")) -> ("Data out"=w654:refnum<class "Data.lvclass">)  [unwired: 9 in]
                }
                frame 214 {
                  # "DTYPE_LIST"
                  n252 = call-dynamic "Get Object Pointer.vi"("Data in"=w660) -> ("Object Pointer"=w656:i64)  [unwired: 8 in, 2 out]
                  n253 = call <vilib>:"Shared Set Object Pointer.vi"("Object Pointer"=w656, "Data in"=refnum<class "Data.lvclass"> refnum ("Data.lvclass")) -> ("Data out"=w659:refnum<class "Data.lvclass">)  [unwired: 9 in]
                }
                frame 215 {
                  # "DTYPE_TUPLE"
                  n254 = call-dynamic "Get Object Pointer.vi"("Data in"=w665) -> ("Object Pointer"=w661:i64)  [unwired: 8 in, 2 out]
                  n255 = call <vilib>:"Shared Set Object Pointer.vi"("Object Pointer"=w661, "Data in"=refnum<class "Data.lvclass"> refnum ("Data.lvclass")) -> ("Data out"=w664:refnum<class "Data.lvclass">)  [unwired: 9 in]
                }
                frame 216 {
                  # "DTYPE_DICTIONARY"
                  n256 = call-dynamic "Get Object Pointer.vi"("Data in"=w670) -> ("Object Pointer"=w666:i64)  [unwired: 8 in, 2 out]
                  n257 = call <vilib>:"Shared Set Object Pointer.vi"("Object Pointer"=w666, "Data in"=refnum<class "Data.lvclass"> refnum ("Data.lvclass")) -> ("Data out"=w669:refnum<class "Data.lvclass">)  [unwired: 9 in]
                }
              }
            }
            frame 4 {
              # "CLASS_A"
              n258 = case shown="0, Default" w675 {
                tunnel: w674 -> [w680 w682 w687 w692 w697 w702 w707 w712 w717 w722 w727 w732 w737 w742 w747 w752 w757 w762 w767 w772 w777 w782 w787 w792 w797 w802 w807 w812 w817 w822 w827 w832 w837 w842 w847 w852 w857 w862 w867 w872 w877 w882]
                tunnel: [w678 w682 w687 w692 w697 w702 w707 w712 w717 w722 w727 w732 w737 w742 w747 w752 w757 w762 w767 w772 w777 w782 w787 w792 w797 w802 w807 w812 w817 w822 w827 w832 w837 w842 w847 w852 w857 w862 w867 w872 w877 w882] -> w673
                tunnel: [w677 w683 w688 w693 w698 w703 w708 w713 w718 w723 w728 w733 w738 w743 w749 w754 w759 w764 w769 w774 w779 w784 w789 w794 w799 w804 w809 w814 w819 w824 w829 w834 w839 w844 w849 w854 w859 w864 w869 w874 w879 w884] -> w671
                tunnel: w672 -> [w677 w685 w689 w694 w699 w704 w709 w714 w719 w724 w729 w734 w739 w744 w750 w755 w760 w765 w770 w775 w780 w785 w790 w795 w800 w805 w810 w815 w820 w825 w830 w835 w840 w845 w850 w855 w860 w865 w870 w875 w880 w885]
                frame 0, Default {
                  n259 = call <vilib>:"Error Cluster From Error Code.vi"("error in (no error)"=w680, "error message (\"\")"="The specified data type does not exist." ("error message (\"\")"), "error code (0)"=42) -> ("error out"=w678:errorcluster)  [unwired: 6 in]
                }
                frame 2 {
                  # "DTYPE_BU"
                  n260 = call-dynamic "Get Object Pointer.vi"("Data in"=w685) -> ("Object Pointer"=w681:i64)  [unwired: 8 in, 2 out]
                  n261 = call <vilib>:"Shared Set Object Pointer.vi"("Object Pointer"=w681, "Data in"=refnum<class "Uint8Array.lvclass"> refnum ("Data.lvclass")) -> ("Data out"=w683:refnum<class "Uint8Array.lvclass">)  [unwired: 9 in]
                }
                frame 3 {
                  # "DTYPE_WU"
                  n262 = call-dynamic "Get Object Pointer.vi"("Data in"=w689) -> ("Object Pointer"=w686:i64)  [unwired: 8 in, 2 out]
                  n263 = call <vilib>:"Shared Set Object Pointer.vi"("Object Pointer"=w686, "Data in"=refnum<class "Uint16Array.lvclass"> refnum ("Data.lvclass")) -> ("Data out"=w688:refnum<class "Uint16Array.lvclass">)  [unwired: 9 in]
                }
                frame 4 {
                  # "DTYPE_LU"
                  n264 = call-dynamic "Get Object Pointer.vi"("Data in"=w694) -> ("Object Pointer"=w691:i64)  [unwired: 8 in, 2 out]
                  n265 = call <vilib>:"Shared Set Object Pointer.vi"("Object Pointer"=w691, "Data in"=refnum<class "Uint32Array.lvclass"> refnum ("Data.lvclass")) -> ("Data out"=w693:refnum<class "Uint32Array.lvclass">)  [unwired: 9 in]
                }
                frame 5 {
                  # "DTYPE_QU"
                  n266 = call-dynamic "Get Object Pointer.vi"("Data in"=w699) -> ("Object Pointer"=w696:i64)  [unwired: 8 in, 2 out]
                  n267 = call <vilib>:"Shared Set Object Pointer.vi"("Object Pointer"=w696, "Data in"=refnum<class "Uint64Array.lvclass"> refnum ("Data.lvclass")) -> ("Data out"=w698:refnum<class "Uint64Array.lvclass">)  [unwired: 9 in]
                }
                frame 6 {
                  # "DTYPE_B"
                  n268 = call-dynamic "Get Object Pointer.vi"("Data in"=w704) -> ("Object Pointer"=w701:i64)  [unwired: 8 in, 2 out]
                  n269 = call <vilib>:"Shared Set Object Pointer.vi"("Object Pointer"=w701, "Data in"=refnum<class "Int8Array.lvclass"> refnum ("Data.lvclass")) -> ("Data out"=w703:refnum<class "Int8Array.lvclass">)  [unwired: 9 in]
                }
                frame 7 {
                  # "DTYPE_W"
                  n270 = call-dynamic "Get Object Pointer.vi"("Data in"=w709) -> ("Object Pointer"=w706:i64)  [unwired: 8 in, 2 out]
                  n271 = call <vilib>:"Shared Set Object Pointer.vi"("Object Pointer"=w706, "Data in"=refnum<class "Int16Array.lvclass"> refnum ("Data.lvclass")) -> ("Data out"=w708:refnum<class "Int16Array.lvclass">)  [unwired: 9 in]
                }
                frame 8 {
                  # "DTYPE_L"
                  n272 = call-dynamic "Get Object Pointer.vi"("Data in"=w714) -> ("Object Pointer"=w711:i64)  [unwired: 8 in, 2 out]
                  n273 = call <vilib>:"Shared Set Object Pointer.vi"("Object Pointer"=w711, "Data in"=refnum<class "Int32Array.lvclass"> refnum ("Data.lvclass")) -> ("Data out"=w713:refnum<class "Int32Array.lvclass">)  [unwired: 9 in]
                }
                frame 9 {
                  # "DTYPE_Q"
                  n274 = call-dynamic "Get Object Pointer.vi"("Data in"=w719) -> ("Object Pointer"=w716:i64)  [unwired: 8 in, 2 out]
                  n275 = call <vilib>:"Shared Set Object Pointer.vi"("Object Pointer"=w716, "Data in"=refnum<class "Int64Array.lvclass"> refnum ("Data.lvclass")) -> ("Data out"=w718:refnum<class "Int64Array.lvclass">)  [unwired: 9 in]
                }
                frame 14 {
                  # "DTYPE_T"
                  n276 = call-dynamic "Get Object Pointer.vi"("Data in"=w724) -> ("Object Pointer"=w721:i64)  [unwired: 8 in, 2 out]
                  n277 = call <vilib>:"Shared Set Object Pointer.vi"("Object Pointer"=w721, "Data in"=refnum<class "StringArray.lvclass"> refnum ("Data.lvclass")) -> ("Data out"=w723:refnum<class "StringArray.lvclass">)  [unwired: 9 in]
                }
                frame 24 {
                  # "DTYPE_DSC"
                  n278 = call-dynamic "Get Object Pointer.vi"("Data in"=w729) -> ("Object Pointer"=w726:i64)  [unwired: 8 in, 2 out]
                  n279 = call <vilib>:"Shared Set Object Pointer.vi"("Object Pointer"=w726, "Data in"=refnum<class "Data.lvclass"> refnum ("Data.lvclass")) -> ("Data out"=w728:refnum<class "Data.lvclass">)  [unwired: 9 in]
                }
                frame 25 {
                  # "DTYPE_OU"
                  n280 = call-dynamic "Get Object Pointer.vi"("Data in"=w734) -> ("Object Pointer"=w731:i64)  [unwired: 8 in, 2 out]
                  n281 = call <vilib>:"Shared Set Object Pointer.vi"("Object Pointer"=w731, "Data in"=refnum<class "Data.lvclass"> refnum ("Data.lvclass")) -> ("Data out"=w733:refnum<class "Data.lvclass">)  [unwired: 9 in]
                }
                frame 26 {
                  # "DTYPE_O"
                  n282 = call-dynamic "Get Object Pointer.vi"("Data in"=w739) -> ("Object Pointer"=w736:i64)  [unwired: 8 in, 2 out]
                  n283 = call <vilib>:"Shared Set Object Pointer.vi"("Object Pointer"=w736, "Data in"=refnum<class "Data.lvclass"> refnum ("Data.lvclass")) -> ("Data out"=w738:refnum<class "Data.lvclass">)  [unwired: 9 in]
                }
                frame 51 {
                  # "DTYPE_POINTER"
                  n284 = call-dynamic "Get Object Pointer.vi"("Data in"=w744) -> ("Object Pointer"=w741:i64)  [unwired: 8 in, 2 out]
                  n285 = call <vilib>:"Shared Set Object Pointer.vi"("Object Pointer"=w741, "Data in"=refnum<class "Data.lvclass"> refnum ("Data.lvclass")) -> ("Data out"=w743:refnum<class "Data.lvclass">)  [unwired: 9 in]
                }
                frame 52 {
                  # "DTYPE_FLOAT"
                  n286 = call-dynamic "Get Object Pointer.vi"("Data in"=w750) -> ("Object Pointer"=w746:i64)  [unwired: 8 in, 2 out]
                  n287 = call <vilib>:"Shared Set Object Pointer.vi"("Object Pointer"=w746, "Data in"=refnum<class "Float32Array.lvclass"> refnum ("Float32Array.lvclass")) -> ("Data out"=w749:refnum<class "Float32Array.lvclass">)  [unwired: 9 in]
                }
                frame 53 {
                  # "DTYPE_DOUBLE"
                  n288 = call-dynamic "Get Object Pointer.vi"("Data in"=w755) -> ("Object Pointer"=w751:i64)  [unwired: 8 in, 2 out]
                  n289 = call <vilib>:"Shared Set Object Pointer.vi"("Object Pointer"=w751, "Data in"=refnum<class "Float64Array.lvclass"> refnum ("Float64Array.lvclass")) -> ("Data out"=w754:refnum<class "Float64Array.lvclass">)  [unwired: 9 in]
                }
                frame 191 {
                  # "DTYPE_IDENT"
                  n290 = call-dynamic "Get Object Pointer.vi"("Data in"=w760) -> ("Object Pointer"=w756:i64)  [unwired: 8 in, 2 out]
                  n291 = call <vilib>:"Shared Set Object Pointer.vi"("Object Pointer"=w756, "Data in"=refnum<class "Data.lvclass"> refnum ("Data.lvclass")) -> ("Data out"=w759:refnum<class "Data.lvclass">)  [unwired: 9 in]
                }
                frame 192 {
                  # "DTYPE_NID"
                  n292 = call-dynamic "Get Object Pointer.vi"("Data in"=w765) -> ("Object Pointer"=w761:i64)  [unwired: 8 in, 2 out]
                  n293 = call <vilib>:"Shared Set Object Pointer.vi"("Object Pointer"=w761, "Data in"=refnum<class "Data.lvclass"> refnum ("Data.lvclass")) -> ("Data out"=w764:refnum<class "Data.lvclass">)  [unwired: 9 in]
                }
                frame 193 {
                  # "DTYPE_PATH"
                  n294 = call-dynamic "Get Object Pointer.vi"("Data in"=w770) -> ("Object Pointer"=w766:i64)  [unwired: 8 in, 2 out]
                  n295 = call <vilib>:"Shared Set Object Pointer.vi"("Object Pointer"=w766, "Data in"=refnum<class "Data.lvclass"> refnum ("Data.lvclass")) -> ("Data out"=w769:refnum<class "Data.lvclass">)  [unwired: 9 in]
                }
                frame 194 {
                  # "DTYPE_PARAM"
                  n296 = call-dynamic "Get Object Pointer.vi"("Data in"=w775) -> ("Object Pointer"=w771:i64)  [unwired: 8 in, 2 out]
                  n297 = call <vilib>:"Shared Set Object Pointer.vi"("Object Pointer"=w771, "Data in"=refnum<class "Data.lvclass"> refnum ("Data.lvclass")) -> ("Data out"=w774:refnum<class "Data.lvclass">)  [unwired: 9 in]
                }
                frame 195 {
                  # "DTYPE_SIGNAL"
                  n298 = call-dynamic "Get Object Pointer.vi"("Data in"=w780) -> ("Object Pointer"=w776:i64)  [unwired: 8 in, 2 out]
                  n299 = call <vilib>:"Shared Set Object Pointer.vi"("Object Pointer"=w776, "Data in"=refnum<class "Data.lvclass"> refnum ("Data.lvclass")) -> ("Data out"=w779:refnum<class "Data.lvclass">)  [unwired: 9 in]
                }
                frame 196 {
                  # "DTYPE_DIMENSION"
                  n300 = call-dynamic "Get Object Pointer.vi"("Data in"=w785) -> ("Object Pointer"=w781:i64)  [unwired: 8 in, 2 out]
                  n301 = call <vilib>:"Shared Set Object Pointer.vi"("Object Pointer"=w781, "Data in"=refnum<class "Data.lvclass"> refnum ("Data.lvclass")) -> ("Data out"=w784:refnum<class "Data.lvclass">)  [unwired: 9 in]
                }
                frame 197 {
                  # "DTYPE_WINDOW"
                  n302 = call-dynamic "Get Object Pointer.vi"("Data in"=w790) -> ("Object Pointer"=w786:i64)  [unwired: 8 in, 2 out]
                  n303 = call <vilib>:"Shared Set Object Pointer.vi"("Object Pointer"=w786, "Data in"=refnum<class "Data.lvclass"> refnum ("Data.lvclass")) -> ("Data out"=w789:refnum<class "Data.lvclass">)  [unwired: 9 in]
                }
                frame 198 {
                  # "DTYPE_SLOPE"
                  n304 = call-dynamic "Get Object Pointer.vi"("Data in"=w795) -> ("Object Pointer"=w791:i64)  [unwired: 8 in, 2 out]
                  n305 = call <vilib>:"Shared Set Object Pointer.vi"("Object Pointer"=w791, "Data in"=refnum<class "Data.lvclass"> refnum ("Data.lvclass")) -> ("Data out"=w794:refnum<class "Data.lvclass">)  [unwired: 9 in]
                }
                frame 199 {
                  # "DTYPE_FUNCTION"
                  n306 = call-dynamic "Get Object Pointer.vi"("Data in"=w800) -> ("Object Pointer"=w796:i64)  [unwired: 8 in, 2 out]
                  n307 = call <vilib>:"Shared Set Object Pointer.vi"("Object Pointer"=w796, "Data in"=refnum<class "Data.lvclass"> refnum ("Data.lvclass")) -> ("Data out"=w799:refnum<class "Data.lvclass">)  [unwired: 9 in]
                }
                frame 200 {
                  # "DTYPE_CONGLOM"
                  n308 = call-dynamic "Get Object Pointer.vi"("Data in"=w805) -> ("Object Pointer"=w801:i64)  [unwired: 8 in, 2 out]
                  n309 = call <vilib>:"Shared Set Object Pointer.vi"("Object Pointer"=w801, "Data in"=refnum<class "Data.lvclass"> refnum ("Data.lvclass")) -> ("Data out"=w804:refnum<class "Data.lvclass">)  [unwired: 9 in]
                }
                frame 201 {
                  # "DTYPE_RANGE"
                  n310 = call-dynamic "Get Object Pointer.vi"("Data in"=w810) -> ("Object Pointer"=w806:i64)  [unwired: 8 in, 2 out]
                  n311 = call <vilib>:"Shared Set Object Pointer.vi"("Object Pointer"=w806, "Data in"=refnum<class "Data.lvclass"> refnum ("Data.lvclass")) -> ("Data out"=w809:refnum<class "Data.lvclass">)  [unwired: 9 in]
                }
                frame 202 {
                  # "DTYPE_ACTION"
                  n312 = call-dynamic "Get Object Pointer.vi"("Data in"=w815) -> ("Object Pointer"=w811:i64)  [unwired: 8 in, 2 out]
                  n313 = call <vilib>:"Shared Set Object Pointer.vi"("Object Pointer"=w811, "Data in"=refnum<class "Data.lvclass"> refnum ("Data.lvclass")) -> ("Data out"=w814:refnum<class "Data.lvclass">)  [unwired: 9 in]
                }
                frame 203 {
                  # "DTYPE_DISPATCH"
                  n314 = call-dynamic "Get Object Pointer.vi"("Data in"=w820) -> ("Object Pointer"=w816:i64)  [unwired: 8 in, 2 out]
                  n315 = call <vilib>:"Shared Set Object Pointer.vi"("Object Pointer"=w816, "Data in"=refnum<class "Data.lvclass"> refnum ("Data.lvclass")) -> ("Data out"=w819:refnum<class "Data.lvclass">)  [unwired: 9 in]
                }
                frame 204 {
                  # "DTYPE_PROGRAM"
                  n316 = call-dynamic "Get Object Pointer.vi"("Data in"=w825) -> ("Object Pointer"=w821:i64)  [unwired: 8 in, 2 out]
                  n317 = call <vilib>:"Shared Set Object Pointer.vi"("Object Pointer"=w821, "Data in"=refnum<class "Data.lvclass"> refnum ("Data.lvclass")) -> ("Data out"=w824:refnum<class "Data.lvclass">)  [unwired: 9 in]
                }
                frame 205 {
                  # "DTYPE_ROUTINE"
                  n318 = call-dynamic "Get Object Pointer.vi"("Data in"=w830) -> ("Object Pointer"=w826:i64)  [unwired: 8 in, 2 out]
                  n319 = call <vilib>:"Shared Set Object Pointer.vi"("Object Pointer"=w826, "Data in"=refnum<class "Data.lvclass"> refnum ("Data.lvclass")) -> ("Data out"=w829:refnum<class "Data.lvclass">)  [unwired: 9 in]
                }
                frame 206 {
                  # "DTYPE_PROCEDURE"
                  n320 = call-dynamic "Get Object Pointer.vi"("Data in"=w835) -> ("Object Pointer"=w831:i64)  [unwired: 8 in, 2 out]
                  n321 = call <vilib>:"Shared Set Object Pointer.vi"("Object Pointer"=w831, "Data in"=refnum<class "Data.lvclass"> refnum ("Data.lvclass")) -> ("Data out"=w834:refnum<class "Data.lvclass">)  [unwired: 9 in]
                }
                frame 207 {
                  # "DTYPE_METHOD"
                  n322 = call-dynamic "Get Object Pointer.vi"("Data in"=w840) -> ("Object Pointer"=w836:i64)  [unwired: 8 in, 2 out]
                  n323 = call <vilib>:"Shared Set Object Pointer.vi"("Object Pointer"=w836, "Data in"=refnum<class "Data.lvclass"> refnum ("Data.lvclass")) -> ("Data out"=w839:refnum<class "Data.lvclass">)  [unwired: 9 in]
                }
                frame 208 {
                  # "DTYPE_DEPENDENCY"
                  n324 = call-dynamic "Get Object Pointer.vi"("Data in"=w845) -> ("Object Pointer"=w841:i64)  [unwired: 8 in, 2 out]
                  n325 = call <vilib>:"Shared Set Object Pointer.vi"("Object Pointer"=w841, "Data in"=refnum<class "Data.lvclass"> refnum ("Data.lvclass")) -> ("Data out"=w844:refnum<class "Data.lvclass">)  [unwired: 9 in]
                }
                frame 209 {
                  # "DTYPE_CONDITION"
                  n326 = call-dynamic "Get Object Pointer.vi"("Data in"=w850) -> ("Object Pointer"=w846:i64)  [unwired: 8 in, 2 out]
                  n327 = call <vilib>:"Shared Set Object Pointer.vi"("Object Pointer"=w846, "Data in"=refnum<class "Data.lvclass"> refnum ("Data.lvclass")) -> ("Data out"=w849:refnum<class "Data.lvclass">)  [unwired: 9 in]
                }
                frame 210 {
                  # "DTYPE_EVENT"
                  n328 = call-dynamic "Get Object Pointer.vi"("Data in"=w855) -> ("Object Pointer"=w851:i64)  [unwired: 8 in, 2 out]
                  n329 = call <vilib>:"Shared Set Object Pointer.vi"("Object Pointer"=w851, "Data in"=refnum<class "Data.lvclass"> refnum ("Data.lvclass")) -> ("Data out"=w854:refnum<class "Data.lvclass">)  [unwired: 9 in]
                }
                frame 211 {
                  # "DTYPE_WITH_UNITS"
                  n330 = call-dynamic "Get Object Pointer.vi"("Data in"=w860) -> ("Object Pointer"=w856:i64)  [unwired: 8 in, 2 out]
                  n331 = call <vilib>:"Shared Set Object Pointer.vi"("Object Pointer"=w856, "Data in"=refnum<class "Data.lvclass"> refnum ("Data.lvclass")) -> ("Data out"=w859:refnum<class "Data.lvclass">)  [unwired: 9 in]
                }
                frame 212 {
                  # "DTYPE_CALL"
                  n332 = call-dynamic "Get Object Pointer.vi"("Data in"=w865) -> ("Object Pointer"=w861:i64)  [unwired: 8 in, 2 out]
                  n333 = call <vilib>:"Shared Set Object Pointer.vi"("Object Pointer"=w861, "Data in"=refnum<class "Data.lvclass"> refnum ("Data.lvclass")) -> ("Data out"=w864:refnum<class "Data.lvclass">)  [unwired: 9 in]
                }
                frame 213 {
                  # "DTYPE_WITH_ERROR"
                  n334 = call-dynamic "Get Object Pointer.vi"("Data in"=w870) -> ("Object Pointer"=w866:i64)  [unwired: 8 in, 2 out]
                  n335 = call <vilib>:"Shared Set Object Pointer.vi"("Object Pointer"=w866, "Data in"=refnum<class "Data.lvclass"> refnum ("Data.lvclass")) -> ("Data out"=w869:refnum<class "Data.lvclass">)  [unwired: 9 in]
                }
                frame 214 {
                  # "DTYPE_LIST"
                  n336 = call-dynamic "Get Object Pointer.vi"("Data in"=w875) -> ("Object Pointer"=w871:i64)  [unwired: 8 in, 2 out]
                  n337 = call <vilib>:"Shared Set Object Pointer.vi"("Object Pointer"=w871, "Data in"=refnum<class "Data.lvclass"> refnum ("Data.lvclass")) -> ("Data out"=w874:refnum<class "Data.lvclass">)  [unwired: 9 in]
                }
                frame 215 {
                  # "DTYPE_TUPLE"
                  n338 = call-dynamic "Get Object Pointer.vi"("Data in"=w880) -> ("Object Pointer"=w876:i64)  [unwired: 8 in, 2 out]
                  n339 = call <vilib>:"Shared Set Object Pointer.vi"("Object Pointer"=w876, "Data in"=refnum<class "Data.lvclass"> refnum ("Data.lvclass")) -> ("Data out"=w879:refnum<class "Data.lvclass">)  [unwired: 9 in]
                }
                frame 216 {
                  # "DTYPE_DICTIONARY"
                  n340 = call-dynamic "Get Object Pointer.vi"("Data in"=w885) -> ("Object Pointer"=w881:i64)  [unwired: 8 in, 2 out]
                  n341 = call <vilib>:"Shared Set Object Pointer.vi"("Object Pointer"=w881, "Data in"=refnum<class "Data.lvclass"> refnum ("Data.lvclass")) -> ("Data out"=w884:refnum<class "Data.lvclass">)  [unwired: 9 in]
                }
              }
            }
            frame 194 {
              # "CLASS_R"
              n342 = case shown="3" w890 {
                tunnel: w889 -> [w895 w897 w902 w907 w912 w917 w922 w927 w932 w937 w942 w947 w952 w957 w962 w967 w972 w977 w982 w987 w992 w997 w1002 w1007 w1012 w1017 w1022 w1027 w1032 w1037 w1042 w1047 w1052 w1057 w1062 w1067 w1072 w1077 w1082 w1087 w1092 w1097]
                tunnel: [w893 w897 w902 w907 w912 w917 w922 w927 w932 w937 w942 w947 w952 w957 w962 w967 w972 w977 w982 w987 w992 w997 w1002 w1007 w1012 w1017 w1022 w1027 w1032 w1037 w1042 w1047 w1052 w1057 w1062 w1067 w1072 w1077 w1082 w1087 w1092 w1097] -> w888
                tunnel: [w892 w898 w903 w908 w913 w918 w923 w928 w933 w938 w943 w948 w953 w958 w964 w969 w974 w979 w984 w989 w994 w999 w1004 w1009 w1014 w1019 w1024 w1029 w1034 w1039 w1044 w1049 w1054 w1059 w1064 w1069 w1074 w1079 w1084 w1089 w1094 w1099] -> w886
                tunnel: w887 -> [w892 w900 w904 w909 w914 w919 w924 w929 w934 w939 w944 w949 w954 w959 w965 w970 w975 w980 w985 w990 w995 w1000 w1005 w1010 w1015 w1020 w1025 w1030 w1035 w1040 w1045 w1050 w1055 w1060 w1065 w1070 w1075 w1080 w1085 w1090 w1095 w1100]
                frame 0, Default {
                  n343 = call <vilib>:"Error Cluster From Error Code.vi"("error in (no error)"=w895, "error message (\"\")"="The specified data type does not exist." ("error message (\"\")"), "error code (0)"=42) -> ("error out"=w893:errorcluster)  [unwired: 6 in]
                }
                frame 2 {
                  # "DTYPE_BU"
                  n344 = call-dynamic "Get Object Pointer.vi"("Data in"=w900) -> ("Object Pointer"=w896:i64)  [unwired: 8 in, 2 out]
                  n345 = call <vilib>:"Shared Set Object Pointer.vi"("Object Pointer"=w896, "Data in"=refnum<class "Data.lvclass"> refnum ("Data.lvclass")) -> ("Data out"=w898:refnum<class "Data.lvclass">)  [unwired: 9 in]
                }
                frame 3 {
                  # "DTYPE_WU"
                  n346 = call-dynamic "Get Object Pointer.vi"("Data in"=w904) -> ("Object Pointer"=w901:i64)  [unwired: 8 in, 2 out]
                  n347 = call <vilib>:"Shared Set Object Pointer.vi"("Object Pointer"=w901, "Data in"=refnum<class "Data.lvclass"> refnum ("Data.lvclass")) -> ("Data out"=w903:refnum<class "Data.lvclass">)  [unwired: 9 in]
                }
                frame 4 {
                  # "DTYPE_LU"
                  n348 = call-dynamic "Get Object Pointer.vi"("Data in"=w909) -> ("Object Pointer"=w906:i64)  [unwired: 8 in, 2 out]
                  n349 = call <vilib>:"Shared Set Object Pointer.vi"("Object Pointer"=w906, "Data in"=refnum<class "Data.lvclass"> refnum ("Data.lvclass")) -> ("Data out"=w908:refnum<class "Data.lvclass">)  [unwired: 9 in]
                }
                frame 5 {
                  # "DTYPE_QU"
                  n350 = call-dynamic "Get Object Pointer.vi"("Data in"=w914) -> ("Object Pointer"=w911:i64)  [unwired: 8 in, 2 out]
                  n351 = call <vilib>:"Shared Set Object Pointer.vi"("Object Pointer"=w911, "Data in"=refnum<class "Data.lvclass"> refnum ("Data.lvclass")) -> ("Data out"=w913:refnum<class "Data.lvclass">)  [unwired: 9 in]
                }
                frame 6 {
                  # "DTYPE_B"
                  n352 = call-dynamic "Get Object Pointer.vi"("Data in"=w919) -> ("Object Pointer"=w916:i64)  [unwired: 8 in, 2 out]
                  n353 = call <vilib>:"Shared Set Object Pointer.vi"("Object Pointer"=w916, "Data in"=refnum<class "Data.lvclass"> refnum ("Data.lvclass")) -> ("Data out"=w918:refnum<class "Data.lvclass">)  [unwired: 9 in]
                }
                frame 7 {
                  # "DTYPE_W"
                  n354 = call-dynamic "Get Object Pointer.vi"("Data in"=w924) -> ("Object Pointer"=w921:i64)  [unwired: 8 in, 2 out]
                  n355 = call <vilib>:"Shared Set Object Pointer.vi"("Object Pointer"=w921, "Data in"=refnum<class "Data.lvclass"> refnum ("Data.lvclass")) -> ("Data out"=w923:refnum<class "Data.lvclass">)  [unwired: 9 in]
                }
                frame 8 {
                  # "DTYPE_L"
                  n356 = call-dynamic "Get Object Pointer.vi"("Data in"=w929) -> ("Object Pointer"=w926:i64)  [unwired: 8 in, 2 out]
                  n357 = call <vilib>:"Shared Set Object Pointer.vi"("Object Pointer"=w926, "Data in"=refnum<class "Data.lvclass"> refnum ("Data.lvclass")) -> ("Data out"=w928:refnum<class "Data.lvclass">)  [unwired: 9 in]
                }
                frame 9 {
                  # "DTYPE_Q"
                  n358 = call-dynamic "Get Object Pointer.vi"("Data in"=w934) -> ("Object Pointer"=w931:i64)  [unwired: 8 in, 2 out]
                  n359 = call <vilib>:"Shared Set Object Pointer.vi"("Object Pointer"=w931, "Data in"=refnum<class "Data.lvclass"> refnum ("Data.lvclass")) -> ("Data out"=w933:refnum<class "Data.lvclass">)  [unwired: 9 in]
                }
                frame 14 {
                  # "DTYPE_T"
                  n360 = call-dynamic "Get Object Pointer.vi"("Data in"=w939) -> ("Object Pointer"=w936:i64)  [unwired: 8 in, 2 out]
                  n361 = call <vilib>:"Shared Set Object Pointer.vi"("Object Pointer"=w936, "Data in"=refnum<class "Data.lvclass"> refnum ("Data.lvclass")) -> ("Data out"=w938:refnum<class "Data.lvclass">)  [unwired: 9 in]
                }
                frame 24 {
                  # "DTYPE_DSC"
                  n362 = call-dynamic "Get Object Pointer.vi"("Data in"=w944) -> ("Object Pointer"=w941:i64)  [unwired: 8 in, 2 out]
                  n363 = call <vilib>:"Shared Set Object Pointer.vi"("Object Pointer"=w941, "Data in"=refnum<class "Data.lvclass"> refnum ("Data.lvclass")) -> ("Data out"=w943:refnum<class "Data.lvclass">)  [unwired: 9 in]
                }
                frame 25 {
                  # "DTYPE_OU"
                  n364 = call-dynamic "Get Object Pointer.vi"("Data in"=w949) -> ("Object Pointer"=w946:i64)  [unwired: 8 in, 2 out]
                  n365 = call <vilib>:"Shared Set Object Pointer.vi"("Object Pointer"=w946, "Data in"=refnum<class "Data.lvclass"> refnum ("Data.lvclass")) -> ("Data out"=w948:refnum<class "Data.lvclass">)  [unwired: 9 in]
                }
                frame 26 {
                  # "DTYPE_O"
                  n366 = call-dynamic "Get Object Pointer.vi"("Data in"=w954) -> ("Object Pointer"=w951:i64)  [unwired: 8 in, 2 out]
                  n367 = call <vilib>:"Shared Set Object Pointer.vi"("Object Pointer"=w951, "Data in"=refnum<class "Data.lvclass"> refnum ("Data.lvclass")) -> ("Data out"=w953:refnum<class "Data.lvclass">)  [unwired: 9 in]
                }
                frame 51 {
                  # "DTYPE_POINTER"
                  n368 = call-dynamic "Get Object Pointer.vi"("Data in"=w959) -> ("Object Pointer"=w956:i64)  [unwired: 8 in, 2 out]
                  n369 = call <vilib>:"Shared Set Object Pointer.vi"("Object Pointer"=w956, "Data in"=refnum<class "Data.lvclass"> refnum ("Data.lvclass")) -> ("Data out"=w958:refnum<class "Data.lvclass">)  [unwired: 9 in]
                }
                frame 52 {
                  # "DTYPE_FLOAT"
                  n370 = call-dynamic "Get Object Pointer.vi"("Data in"=w965) -> ("Object Pointer"=w961:i64)  [unwired: 8 in, 2 out]
                  n371 = call <vilib>:"Shared Set Object Pointer.vi"("Object Pointer"=w961, "Data in"=refnum<class "Data.lvclass"> refnum ("Data.lvclass")) -> ("Data out"=w964:refnum<class "Data.lvclass">)  [unwired: 9 in]
                }
                frame 53 {
                  # "DTYPE_DOUBLE"
                  n372 = call-dynamic "Get Object Pointer.vi"("Data in"=w970) -> ("Object Pointer"=w966:i64)  [unwired: 8 in, 2 out]
                  n373 = call <vilib>:"Shared Set Object Pointer.vi"("Object Pointer"=w966, "Data in"=refnum<class "Data.lvclass"> refnum ("Data.lvclass")) -> ("Data out"=w969:refnum<class "Data.lvclass">)  [unwired: 9 in]
                }
                frame 191 {
                  # "DTYPE_IDENT"
                  n374 = call-dynamic "Get Object Pointer.vi"("Data in"=w975) -> ("Object Pointer"=w971:i64)  [unwired: 8 in, 2 out]
                  n375 = call <vilib>:"Shared Set Object Pointer.vi"("Object Pointer"=w971, "Data in"=refnum<class "Data.lvclass"> refnum ("Data.lvclass")) -> ("Data out"=w974:refnum<class "Data.lvclass">)  [unwired: 9 in]
                }
                frame 192 {
                  # "DTYPE_NID"
                  n376 = call-dynamic "Get Object Pointer.vi"("Data in"=w980) -> ("Object Pointer"=w976:i64)  [unwired: 8 in, 2 out]
                  n377 = call <vilib>:"Shared Set Object Pointer.vi"("Object Pointer"=w976, "Data in"=refnum<class "Data.lvclass"> refnum ("Data.lvclass")) -> ("Data out"=w979:refnum<class "Data.lvclass">)  [unwired: 9 in]
                }
                frame 193 {
                  # "DTYPE_PATH"
                  n378 = call-dynamic "Get Object Pointer.vi"("Data in"=w985) -> ("Object Pointer"=w981:i64)  [unwired: 8 in, 2 out]
                  n379 = call <vilib>:"Shared Set Object Pointer.vi"("Object Pointer"=w981, "Data in"=refnum<class "Data.lvclass"> refnum ("Data.lvclass")) -> ("Data out"=w984:refnum<class "Data.lvclass">)  [unwired: 9 in]
                }
                frame 194 {
                  # "DTYPE_PARAM"
                  n380 = call-dynamic "Get Object Pointer.vi"("Data in"=w990) -> ("Object Pointer"=w986:i64)  [unwired: 8 in, 2 out]
                  n381 = call <vilib>:"Shared Set Object Pointer.vi"("Object Pointer"=w986, "Data in"=refnum<class "Data.lvclass"> refnum ("Data.lvclass")) -> ("Data out"=w989:refnum<class "Data.lvclass">)  [unwired: 9 in]
                }
                frame 195 {
                  # "DTYPE_SIGNAL"
                  n382 = call-dynamic "Get Object Pointer.vi"("Data in"=w995) -> ("Object Pointer"=w991:i64)  [unwired: 8 in, 2 out]
                  n383 = call <vilib>:"Shared Set Object Pointer.vi"("Object Pointer"=w991, "Data in"=refnum<class "Data.lvclass"> refnum ("Data.lvclass")) -> ("Data out"=w994:refnum<class "Data.lvclass">)  [unwired: 9 in]
                }
                frame 196 {
                  # "DTYPE_DIMENSION"
                  n384 = call-dynamic "Get Object Pointer.vi"("Data in"=w1000) -> ("Object Pointer"=w996:i64)  [unwired: 8 in, 2 out]
                  n385 = call <vilib>:"Shared Set Object Pointer.vi"("Object Pointer"=w996, "Data in"=refnum<class "Data.lvclass"> refnum ("Data.lvclass")) -> ("Data out"=w999:refnum<class "Data.lvclass">)  [unwired: 9 in]
                }
                frame 197 {
                  # "DTYPE_WINDOW"
                  n386 = call-dynamic "Get Object Pointer.vi"("Data in"=w1005) -> ("Object Pointer"=w1001:i64)  [unwired: 8 in, 2 out]
                  n387 = call <vilib>:"Shared Set Object Pointer.vi"("Object Pointer"=w1001, "Data in"=refnum<class "Data.lvclass"> refnum ("Data.lvclass")) -> ("Data out"=w1004:refnum<class "Data.lvclass">)  [unwired: 9 in]
                }
                frame 198 {
                  # "DTYPE_SLOPE"
                  n388 = call-dynamic "Get Object Pointer.vi"("Data in"=w1010) -> ("Object Pointer"=w1006:i64)  [unwired: 8 in, 2 out]
                  n389 = call <vilib>:"Shared Set Object Pointer.vi"("Object Pointer"=w1006, "Data in"=refnum<class "Data.lvclass"> refnum ("Data.lvclass")) -> ("Data out"=w1009:refnum<class "Data.lvclass">)  [unwired: 9 in]
                }
                frame 199 {
                  # "DTYPE_FUNCTION"
                  n390 = call-dynamic "Get Object Pointer.vi"("Data in"=w1015) -> ("Object Pointer"=w1011:i64)  [unwired: 8 in, 2 out]
                  n391 = call <vilib>:"Shared Set Object Pointer.vi"("Object Pointer"=w1011, "Data in"=refnum<class "Data.lvclass"> refnum ("Data.lvclass")) -> ("Data out"=w1014:refnum<class "Data.lvclass">)  [unwired: 9 in]
                }
                frame 200 {
                  # "DTYPE_CONGLOM"
                  n392 = call-dynamic "Get Object Pointer.vi"("Data in"=w1020) -> ("Object Pointer"=w1016:i64)  [unwired: 8 in, 2 out]
                  n393 = call <vilib>:"Shared Set Object Pointer.vi"("Object Pointer"=w1016, "Data in"=refnum<class "Data.lvclass"> refnum ("Data.lvclass")) -> ("Data out"=w1019:refnum<class "Data.lvclass">)  [unwired: 9 in]
                }
                frame 201 {
                  # "DTYPE_RANGE"
                  n394 = call-dynamic "Get Object Pointer.vi"("Data in"=w1025) -> ("Object Pointer"=w1021:i64)  [unwired: 8 in, 2 out]
                  n395 = call <vilib>:"Shared Set Object Pointer.vi"("Object Pointer"=w1021, "Data in"=refnum<class "Data.lvclass"> refnum ("Data.lvclass")) -> ("Data out"=w1024:refnum<class "Data.lvclass">)  [unwired: 9 in]
                }
                frame 202 {
                  # "DTYPE_ACTION"
                  n396 = call-dynamic "Get Object Pointer.vi"("Data in"=w1030) -> ("Object Pointer"=w1026:i64)  [unwired: 8 in, 2 out]
                  n397 = call <vilib>:"Shared Set Object Pointer.vi"("Object Pointer"=w1026, "Data in"=refnum<class "Data.lvclass"> refnum ("Data.lvclass")) -> ("Data out"=w1029:refnum<class "Data.lvclass">)  [unwired: 9 in]
                }
                frame 203 {
                  # "DTYPE_DISPATCH"
                  n398 = call-dynamic "Get Object Pointer.vi"("Data in"=w1035) -> ("Object Pointer"=w1031:i64)  [unwired: 8 in, 2 out]
                  n399 = call <vilib>:"Shared Set Object Pointer.vi"("Object Pointer"=w1031, "Data in"=refnum<class "Data.lvclass"> refnum ("Data.lvclass")) -> ("Data out"=w1034:refnum<class "Data.lvclass">)  [unwired: 9 in]
                }
                frame 204 {
                  # "DTYPE_PROGRAM"
                  n400 = call-dynamic "Get Object Pointer.vi"("Data in"=w1040) -> ("Object Pointer"=w1036:i64)  [unwired: 8 in, 2 out]
                  n401 = call <vilib>:"Shared Set Object Pointer.vi"("Object Pointer"=w1036, "Data in"=refnum<class "Data.lvclass"> refnum ("Data.lvclass")) -> ("Data out"=w1039:refnum<class "Data.lvclass">)  [unwired: 9 in]
                }
                frame 205 {
                  # "DTYPE_ROUTINE"
                  n402 = call-dynamic "Get Object Pointer.vi"("Data in"=w1045) -> ("Object Pointer"=w1041:i64)  [unwired: 8 in, 2 out]
                  n403 = call <vilib>:"Shared Set Object Pointer.vi"("Object Pointer"=w1041, "Data in"=refnum<class "Data.lvclass"> refnum ("Data.lvclass")) -> ("Data out"=w1044:refnum<class "Data.lvclass">)  [unwired: 9 in]
                }
                frame 206 {
                  # "DTYPE_PROCEDURE"
                  n404 = call-dynamic "Get Object Pointer.vi"("Data in"=w1050) -> ("Object Pointer"=w1046:i64)  [unwired: 8 in, 2 out]
                  n405 = call <vilib>:"Shared Set Object Pointer.vi"("Object Pointer"=w1046, "Data in"=refnum<class "Data.lvclass"> refnum ("Data.lvclass")) -> ("Data out"=w1049:refnum<class "Data.lvclass">)  [unwired: 9 in]
                }
                frame 207 {
                  # "DTYPE_METHOD"
                  n406 = call-dynamic "Get Object Pointer.vi"("Data in"=w1055) -> ("Object Pointer"=w1051:i64)  [unwired: 8 in, 2 out]
                  n407 = call <vilib>:"Shared Set Object Pointer.vi"("Object Pointer"=w1051, "Data in"=refnum<class "Data.lvclass"> refnum ("Data.lvclass")) -> ("Data out"=w1054:refnum<class "Data.lvclass">)  [unwired: 9 in]
                }
                frame 208 {
                  # "DTYPE_DEPENDENCY"
                  n408 = call-dynamic "Get Object Pointer.vi"("Data in"=w1060) -> ("Object Pointer"=w1056:i64)  [unwired: 8 in, 2 out]
                  n409 = call <vilib>:"Shared Set Object Pointer.vi"("Object Pointer"=w1056, "Data in"=refnum<class "Data.lvclass"> refnum ("Data.lvclass")) -> ("Data out"=w1059:refnum<class "Data.lvclass">)  [unwired: 9 in]
                }
                frame 209 {
                  # "DTYPE_CONDITION"
                  n410 = call-dynamic "Get Object Pointer.vi"("Data in"=w1065) -> ("Object Pointer"=w1061:i64)  [unwired: 8 in, 2 out]
                  n411 = call <vilib>:"Shared Set Object Pointer.vi"("Object Pointer"=w1061, "Data in"=refnum<class "Data.lvclass"> refnum ("Data.lvclass")) -> ("Data out"=w1064:refnum<class "Data.lvclass">)  [unwired: 9 in]
                }
                frame 210 {
                  # "DTYPE_EVENT"
                  n412 = call-dynamic "Get Object Pointer.vi"("Data in"=w1070) -> ("Object Pointer"=w1066:i64)  [unwired: 8 in, 2 out]
                  n413 = call <vilib>:"Shared Set Object Pointer.vi"("Object Pointer"=w1066, "Data in"=refnum<class "Data.lvclass"> refnum ("Data.lvclass")) -> ("Data out"=w1069:refnum<class "Data.lvclass">)  [unwired: 9 in]
                }
                frame 211 {
                  # "DTYPE_WITH_UNITS"
                  n414 = call-dynamic "Get Object Pointer.vi"("Data in"=w1075) -> ("Object Pointer"=w1071:i64)  [unwired: 8 in, 2 out]
                  n415 = call <vilib>:"Shared Set Object Pointer.vi"("Object Pointer"=w1071, "Data in"=refnum<class "Data.lvclass"> refnum ("Data.lvclass")) -> ("Data out"=w1074:refnum<class "Data.lvclass">)  [unwired: 9 in]
                }
                frame 212 {
                  # "DTYPE_CALL"
                  n416 = call-dynamic "Get Object Pointer.vi"("Data in"=w1080) -> ("Object Pointer"=w1076:i64)  [unwired: 8 in, 2 out]
                  n417 = call <vilib>:"Shared Set Object Pointer.vi"("Object Pointer"=w1076, "Data in"=refnum<class "Data.lvclass"> refnum ("Data.lvclass")) -> ("Data out"=w1079:refnum<class "Data.lvclass">)  [unwired: 9 in]
                }
                frame 213 {
                  # "DTYPE_WITH_ERROR"
                  n418 = call-dynamic "Get Object Pointer.vi"("Data in"=w1085) -> ("Object Pointer"=w1081:i64)  [unwired: 8 in, 2 out]
                  n419 = call <vilib>:"Shared Set Object Pointer.vi"("Object Pointer"=w1081, "Data in"=refnum<class "Data.lvclass"> refnum ("Data.lvclass")) -> ("Data out"=w1084:refnum<class "Data.lvclass">)  [unwired: 9 in]
                }
                frame 214 {
                  # "DTYPE_LIST"
                  n420 = call-dynamic "Get Object Pointer.vi"("Data in"=w1090) -> ("Object Pointer"=w1086:i64)  [unwired: 8 in, 2 out]
                  n421 = call <vilib>:"Shared Set Object Pointer.vi"("Object Pointer"=w1086, "Data in"=refnum<class "Data.lvclass"> refnum ("Data.lvclass")) -> ("Data out"=w1089:refnum<class "Data.lvclass">)  [unwired: 9 in]
                }
                frame 215 {
                  # "DTYPE_TUPLE"
                  n422 = call-dynamic "Get Object Pointer.vi"("Data in"=w1095) -> ("Object Pointer"=w1091:i64)  [unwired: 8 in, 2 out]
                  n423 = call <vilib>:"Shared Set Object Pointer.vi"("Object Pointer"=w1091, "Data in"=refnum<class "Data.lvclass"> refnum ("Data.lvclass")) -> ("Data out"=w1094:refnum<class "Data.lvclass">)  [unwired: 9 in]
                }
                frame 216 {
                  # "DTYPE_DICTIONARY"
                  n424 = call-dynamic "Get Object Pointer.vi"("Data in"=w1100) -> ("Object Pointer"=w1096:i64)  [unwired: 8 in, 2 out]
                  n425 = call <vilib>:"Shared Set Object Pointer.vi"("Object Pointer"=w1096, "Data in"=refnum<class "Data.lvclass"> refnum ("Data.lvclass")) -> ("Data out"=w1099:refnum<class "Data.lvclass">)  [unwired: 9 in]
                }
              }
            }
            frame 196 {
              # "CLASS_APD"
              n426 = case shown="0, Default" w1105 {
                tunnel: w1104 -> [w1110 w1112 w1117 w1122 w1127 w1132 w1137 w1142 w1147 w1152 w1157 w1162 w1167 w1172 w1177 w1182 w1187 w1192 w1197 w1202 w1207 w1212 w1217 w1222 w1227 w1232 w1237 w1242 w1247 w1252 w1257 w1262 w1267 w1272 w1277 w1282 w1287 w1292 w1297 w1302 w1307 w1312]
                tunnel: [w1108 w1112 w1117 w1122 w1127 w1132 w1137 w1142 w1147 w1152 w1157 w1162 w1167 w1172 w1177 w1182 w1187 w1192 w1197 w1202 w1207 w1212 w1217 w1222 w1227 w1232 w1237 w1242 w1247 w1252 w1257 w1262 w1267 w1272 w1277 w1282 w1287 w1292 w1297 w1302 w1307 w1312] -> w1103
                tunnel: [w1107 w1113 w1118 w1123 w1128 w1133 w1138 w1143 w1148 w1153 w1158 w1163 w1168 w1173 w1179 w1184 w1189 w1194 w1199 w1204 w1209 w1214 w1219 w1224 w1229 w1234 w1239 w1244 w1249 w1254 w1259 w1264 w1269 w1274 w1279 w1284 w1289 w1294 w1299 w1304 w1309 w1314] -> w1101
                tunnel: w1102 -> [w1107 w1115 w1119 w1124 w1129 w1134 w1139 w1144 w1149 w1154 w1159 w1164 w1169 w1174 w1180 w1185 w1190 w1195 w1200 w1205 w1210 w1215 w1220 w1225 w1230 w1235 w1240 w1245 w1250 w1255 w1260 w1265 w1270 w1275 w1280 w1285 w1290 w1295 w1300 w1305 w1310 w1315]
                frame 0, Default {
                  n427 = call <vilib>:"Error Cluster From Error Code.vi"("error in (no error)"=w1110, "error message (\"\")"="The specified data type does not exist." ("error message (\"\")"), "error code (0)"=42) -> ("error out"=w1108:errorcluster)  [unwired: 6 in]
                }
                frame 2 {
                  # "DTYPE_BU"
                  n428 = call-dynamic "Get Object Pointer.vi"("Data in"=w1115) -> ("Object Pointer"=w1111:i64)  [unwired: 8 in, 2 out]
                  n429 = call <vilib>:"Shared Set Object Pointer.vi"("Object Pointer"=w1111, "Data in"=refnum<class "Data.lvclass"> refnum ("Data.lvclass")) -> ("Data out"=w1113:refnum<class "Data.lvclass">)  [unwired: 9 in]
                }
                frame 3 {
                  # "DTYPE_WU"
                  n430 = call-dynamic "Get Object Pointer.vi"("Data in"=w1119) -> ("Object Pointer"=w1116:i64)  [unwired: 8 in, 2 out]
                  n431 = call <vilib>:"Shared Set Object Pointer.vi"("Object Pointer"=w1116, "Data in"=refnum<class "Data.lvclass"> refnum ("Data.lvclass")) -> ("Data out"=w1118:refnum<class "Data.lvclass">)  [unwired: 9 in]
                }
                frame 4 {
                  # "DTYPE_LU"
                  n432 = call-dynamic "Get Object Pointer.vi"("Data in"=w1124) -> ("Object Pointer"=w1121:i64)  [unwired: 8 in, 2 out]
                  n433 = call <vilib>:"Shared Set Object Pointer.vi"("Object Pointer"=w1121, "Data in"=refnum<class "Data.lvclass"> refnum ("Data.lvclass")) -> ("Data out"=w1123:refnum<class "Data.lvclass">)  [unwired: 9 in]
                }
                frame 5 {
                  # "DTYPE_QU"
                  n434 = call-dynamic "Get Object Pointer.vi"("Data in"=w1129) -> ("Object Pointer"=w1126:i64)  [unwired: 8 in, 2 out]
                  n435 = call <vilib>:"Shared Set Object Pointer.vi"("Object Pointer"=w1126, "Data in"=refnum<class "Data.lvclass"> refnum ("Data.lvclass")) -> ("Data out"=w1128:refnum<class "Data.lvclass">)  [unwired: 9 in]
                }
                frame 6 {
                  # "DTYPE_B"
                  n436 = call-dynamic "Get Object Pointer.vi"("Data in"=w1134) -> ("Object Pointer"=w1131:i64)  [unwired: 8 in, 2 out]
                  n437 = call <vilib>:"Shared Set Object Pointer.vi"("Object Pointer"=w1131, "Data in"=refnum<class "Data.lvclass"> refnum ("Data.lvclass")) -> ("Data out"=w1133:refnum<class "Data.lvclass">)  [unwired: 9 in]
                }
                frame 7 {
                  # "DTYPE_W"
                  n438 = call-dynamic "Get Object Pointer.vi"("Data in"=w1139) -> ("Object Pointer"=w1136:i64)  [unwired: 8 in, 2 out]
                  n439 = call <vilib>:"Shared Set Object Pointer.vi"("Object Pointer"=w1136, "Data in"=refnum<class "Data.lvclass"> refnum ("Data.lvclass")) -> ("Data out"=w1138:refnum<class "Data.lvclass">)  [unwired: 9 in]
                }
                frame 8 {
                  # "DTYPE_L"
                  n440 = call-dynamic "Get Object Pointer.vi"("Data in"=w1144) -> ("Object Pointer"=w1141:i64)  [unwired: 8 in, 2 out]
                  n441 = call <vilib>:"Shared Set Object Pointer.vi"("Object Pointer"=w1141, "Data in"=refnum<class "Data.lvclass"> refnum ("Data.lvclass")) -> ("Data out"=w1143:refnum<class "Data.lvclass">)  [unwired: 9 in]
                }
                frame 9 {
                  # "DTYPE_Q"
                  n442 = call-dynamic "Get Object Pointer.vi"("Data in"=w1149) -> ("Object Pointer"=w1146:i64)  [unwired: 8 in, 2 out]
                  n443 = call <vilib>:"Shared Set Object Pointer.vi"("Object Pointer"=w1146, "Data in"=refnum<class "Data.lvclass"> refnum ("Data.lvclass")) -> ("Data out"=w1148:refnum<class "Data.lvclass">)  [unwired: 9 in]
                }
                frame 14 {
                  # "DTYPE_T"
                  n444 = call-dynamic "Get Object Pointer.vi"("Data in"=w1154) -> ("Object Pointer"=w1151:i64)  [unwired: 8 in, 2 out]
                  n445 = call <vilib>:"Shared Set Object Pointer.vi"("Object Pointer"=w1151, "Data in"=refnum<class "Data.lvclass"> refnum ("Data.lvclass")) -> ("Data out"=w1153:refnum<class "Data.lvclass">)  [unwired: 9 in]
                }
                frame 24 {
                  # "DTYPE_DSC"
                  n446 = call-dynamic "Get Object Pointer.vi"("Data in"=w1159) -> ("Object Pointer"=w1156:i64)  [unwired: 8 in, 2 out]
                  n447 = call <vilib>:"Shared Set Object Pointer.vi"("Object Pointer"=w1156, "Data in"=refnum<class "Data.lvclass"> refnum ("Data.lvclass")) -> ("Data out"=w1158:refnum<class "Data.lvclass">)  [unwired: 9 in]
                }
                frame 25 {
                  # "DTYPE_OU"
                  n448 = call-dynamic "Get Object Pointer.vi"("Data in"=w1164) -> ("Object Pointer"=w1161:i64)  [unwired: 8 in, 2 out]
                  n449 = call <vilib>:"Shared Set Object Pointer.vi"("Object Pointer"=w1161, "Data in"=refnum<class "Data.lvclass"> refnum ("Data.lvclass")) -> ("Data out"=w1163:refnum<class "Data.lvclass">)  [unwired: 9 in]
                }
                frame 26 {
                  # "DTYPE_O"
                  n450 = call-dynamic "Get Object Pointer.vi"("Data in"=w1169) -> ("Object Pointer"=w1166:i64)  [unwired: 8 in, 2 out]
                  n451 = call <vilib>:"Shared Set Object Pointer.vi"("Object Pointer"=w1166, "Data in"=refnum<class "Data.lvclass"> refnum ("Data.lvclass")) -> ("Data out"=w1168:refnum<class "Data.lvclass">)  [unwired: 9 in]
                }
                frame 51 {
                  # "DTYPE_POINTER"
                  n452 = call-dynamic "Get Object Pointer.vi"("Data in"=w1174) -> ("Object Pointer"=w1171:i64)  [unwired: 8 in, 2 out]
                  n453 = call <vilib>:"Shared Set Object Pointer.vi"("Object Pointer"=w1171, "Data in"=refnum<class "Data.lvclass"> refnum ("Data.lvclass")) -> ("Data out"=w1173:refnum<class "Data.lvclass">)  [unwired: 9 in]
                }
                frame 52 {
                  # "DTYPE_FLOAT"
                  n454 = call-dynamic "Get Object Pointer.vi"("Data in"=w1180) -> ("Object Pointer"=w1176:i64)  [unwired: 8 in, 2 out]
                  n455 = call <vilib>:"Shared Set Object Pointer.vi"("Object Pointer"=w1176, "Data in"=refnum<class "Data.lvclass"> refnum ("Data.lvclass")) -> ("Data out"=w1179:refnum<class "Data.lvclass">)  [unwired: 9 in]
                }
                frame 53 {
                  # "DTYPE_DOUBLE"
                  n456 = call-dynamic "Get Object Pointer.vi"("Data in"=w1185) -> ("Object Pointer"=w1181:i64)  [unwired: 8 in, 2 out]
                  n457 = call <vilib>:"Shared Set Object Pointer.vi"("Object Pointer"=w1181, "Data in"=refnum<class "Data.lvclass"> refnum ("Data.lvclass")) -> ("Data out"=w1184:refnum<class "Data.lvclass">)  [unwired: 9 in]
                }
                frame 191 {
                  # "DTYPE_IDENT"
                  n458 = call-dynamic "Get Object Pointer.vi"("Data in"=w1190) -> ("Object Pointer"=w1186:i64)  [unwired: 8 in, 2 out]
                  n459 = call <vilib>:"Shared Set Object Pointer.vi"("Object Pointer"=w1186, "Data in"=refnum<class "Data.lvclass"> refnum ("Data.lvclass")) -> ("Data out"=w1189:refnum<class "Data.lvclass">)  [unwired: 9 in]
                }
                frame 192 {
                  # "DTYPE_NID"
                  n460 = call-dynamic "Get Object Pointer.vi"("Data in"=w1195) -> ("Object Pointer"=w1191:i64)  [unwired: 8 in, 2 out]
                  n461 = call <vilib>:"Shared Set Object Pointer.vi"("Object Pointer"=w1191, "Data in"=refnum<class "Data.lvclass"> refnum ("Data.lvclass")) -> ("Data out"=w1194:refnum<class "Data.lvclass">)  [unwired: 9 in]
                }
                frame 193 {
                  # "DTYPE_PATH"
                  n462 = call-dynamic "Get Object Pointer.vi"("Data in"=w1200) -> ("Object Pointer"=w1196:i64)  [unwired: 8 in, 2 out]
                  n463 = call <vilib>:"Shared Set Object Pointer.vi"("Object Pointer"=w1196, "Data in"=refnum<class "Data.lvclass"> refnum ("Data.lvclass")) -> ("Data out"=w1199:refnum<class "Data.lvclass">)  [unwired: 9 in]
                }
                frame 194 {
                  # "DTYPE_PARAM"
                  n464 = call-dynamic "Get Object Pointer.vi"("Data in"=w1205) -> ("Object Pointer"=w1201:i64)  [unwired: 8 in, 2 out]
                  n465 = call <vilib>:"Shared Set Object Pointer.vi"("Object Pointer"=w1201, "Data in"=refnum<class "Data.lvclass"> refnum ("Data.lvclass")) -> ("Data out"=w1204:refnum<class "Data.lvclass">)  [unwired: 9 in]
                }
                frame 195 {
                  # "DTYPE_SIGNAL"
                  n466 = call-dynamic "Get Object Pointer.vi"("Data in"=w1210) -> ("Object Pointer"=w1206:i64)  [unwired: 8 in, 2 out]
                  n467 = call <vilib>:"Shared Set Object Pointer.vi"("Object Pointer"=w1206, "Data in"=refnum<class "Data.lvclass"> refnum ("Data.lvclass")) -> ("Data out"=w1209:refnum<class "Data.lvclass">)  [unwired: 9 in]
                }
                frame 196 {
                  # "DTYPE_DIMENSION"
                  n468 = call-dynamic "Get Object Pointer.vi"("Data in"=w1215) -> ("Object Pointer"=w1211:i64)  [unwired: 8 in, 2 out]
                  n469 = call <vilib>:"Shared Set Object Pointer.vi"("Object Pointer"=w1211, "Data in"=refnum<class "Data.lvclass"> refnum ("Data.lvclass")) -> ("Data out"=w1214:refnum<class "Data.lvclass">)  [unwired: 9 in]
                }
                frame 197 {
                  # "DTYPE_WINDOW"
                  n470 = call-dynamic "Get Object Pointer.vi"("Data in"=w1220) -> ("Object Pointer"=w1216:i64)  [unwired: 8 in, 2 out]
                  n471 = call <vilib>:"Shared Set Object Pointer.vi"("Object Pointer"=w1216, "Data in"=refnum<class "Data.lvclass"> refnum ("Data.lvclass")) -> ("Data out"=w1219:refnum<class "Data.lvclass">)  [unwired: 9 in]
                }
                frame 198 {
                  # "DTYPE_SLOPE"
                  n472 = call-dynamic "Get Object Pointer.vi"("Data in"=w1225) -> ("Object Pointer"=w1221:i64)  [unwired: 8 in, 2 out]
                  n473 = call <vilib>:"Shared Set Object Pointer.vi"("Object Pointer"=w1221, "Data in"=refnum<class "Data.lvclass"> refnum ("Data.lvclass")) -> ("Data out"=w1224:refnum<class "Data.lvclass">)  [unwired: 9 in]
                }
                frame 199 {
                  # "DTYPE_FUNCTION"
                  n474 = call-dynamic "Get Object Pointer.vi"("Data in"=w1230) -> ("Object Pointer"=w1226:i64)  [unwired: 8 in, 2 out]
                  n475 = call <vilib>:"Shared Set Object Pointer.vi"("Object Pointer"=w1226, "Data in"=refnum<class "Data.lvclass"> refnum ("Data.lvclass")) -> ("Data out"=w1229:refnum<class "Data.lvclass">)  [unwired: 9 in]
                }
                frame 200 {
                  # "DTYPE_CONGLOM"
                  n476 = call-dynamic "Get Object Pointer.vi"("Data in"=w1235) -> ("Object Pointer"=w1231:i64)  [unwired: 8 in, 2 out]
                  n477 = call <vilib>:"Shared Set Object Pointer.vi"("Object Pointer"=w1231, "Data in"=refnum<class "Data.lvclass"> refnum ("Data.lvclass")) -> ("Data out"=w1234:refnum<class "Data.lvclass">)  [unwired: 9 in]
                }
                frame 201 {
                  # "DTYPE_RANGE"
                  n478 = call-dynamic "Get Object Pointer.vi"("Data in"=w1240) -> ("Object Pointer"=w1236:i64)  [unwired: 8 in, 2 out]
                  n479 = call <vilib>:"Shared Set Object Pointer.vi"("Object Pointer"=w1236, "Data in"=refnum<class "Data.lvclass"> refnum ("Data.lvclass")) -> ("Data out"=w1239:refnum<class "Data.lvclass">)  [unwired: 9 in]
                }
                frame 202 {
                  # "DTYPE_ACTION"
                  n480 = call-dynamic "Get Object Pointer.vi"("Data in"=w1245) -> ("Object Pointer"=w1241:i64)  [unwired: 8 in, 2 out]
                  n481 = call <vilib>:"Shared Set Object Pointer.vi"("Object Pointer"=w1241, "Data in"=refnum<class "Data.lvclass"> refnum ("Data.lvclass")) -> ("Data out"=w1244:refnum<class "Data.lvclass">)  [unwired: 9 in]
                }
                frame 203 {
                  # "DTYPE_DISPATCH"
                  n482 = call-dynamic "Get Object Pointer.vi"("Data in"=w1250) -> ("Object Pointer"=w1246:i64)  [unwired: 8 in, 2 out]
                  n483 = call <vilib>:"Shared Set Object Pointer.vi"("Object Pointer"=w1246, "Data in"=refnum<class "Data.lvclass"> refnum ("Data.lvclass")) -> ("Data out"=w1249:refnum<class "Data.lvclass">)  [unwired: 9 in]
                }
                frame 204 {
                  # "DTYPE_PROGRAM"
                  n484 = call-dynamic "Get Object Pointer.vi"("Data in"=w1255) -> ("Object Pointer"=w1251:i64)  [unwired: 8 in, 2 out]
                  n485 = call <vilib>:"Shared Set Object Pointer.vi"("Object Pointer"=w1251, "Data in"=refnum<class "Data.lvclass"> refnum ("Data.lvclass")) -> ("Data out"=w1254:refnum<class "Data.lvclass">)  [unwired: 9 in]
                }
                frame 205 {
                  # "DTYPE_ROUTINE"
                  n486 = call-dynamic "Get Object Pointer.vi"("Data in"=w1260) -> ("Object Pointer"=w1256:i64)  [unwired: 8 in, 2 out]
                  n487 = call <vilib>:"Shared Set Object Pointer.vi"("Object Pointer"=w1256, "Data in"=refnum<class "Data.lvclass"> refnum ("Data.lvclass")) -> ("Data out"=w1259:refnum<class "Data.lvclass">)  [unwired: 9 in]
                }
                frame 206 {
                  # "DTYPE_PROCEDURE"
                  n488 = call-dynamic "Get Object Pointer.vi"("Data in"=w1265) -> ("Object Pointer"=w1261:i64)  [unwired: 8 in, 2 out]
                  n489 = call <vilib>:"Shared Set Object Pointer.vi"("Object Pointer"=w1261, "Data in"=refnum<class "Data.lvclass"> refnum ("Data.lvclass")) -> ("Data out"=w1264:refnum<class "Data.lvclass">)  [unwired: 9 in]
                }
                frame 207 {
                  # "DTYPE_METHOD"
                  n490 = call-dynamic "Get Object Pointer.vi"("Data in"=w1270) -> ("Object Pointer"=w1266:i64)  [unwired: 8 in, 2 out]
                  n491 = call <vilib>:"Shared Set Object Pointer.vi"("Object Pointer"=w1266, "Data in"=refnum<class "Data.lvclass"> refnum ("Data.lvclass")) -> ("Data out"=w1269:refnum<class "Data.lvclass">)  [unwired: 9 in]
                }
                frame 208 {
                  # "DTYPE_DEPENDENCY"
                  n492 = call-dynamic "Get Object Pointer.vi"("Data in"=w1275) -> ("Object Pointer"=w1271:i64)  [unwired: 8 in, 2 out]
                  n493 = call <vilib>:"Shared Set Object Pointer.vi"("Object Pointer"=w1271, "Data in"=refnum<class "Data.lvclass"> refnum ("Data.lvclass")) -> ("Data out"=w1274:refnum<class "Data.lvclass">)  [unwired: 9 in]
                }
                frame 209 {
                  # "DTYPE_CONDITION"
                  n494 = call-dynamic "Get Object Pointer.vi"("Data in"=w1280) -> ("Object Pointer"=w1276:i64)  [unwired: 8 in, 2 out]
                  n495 = call <vilib>:"Shared Set Object Pointer.vi"("Object Pointer"=w1276, "Data in"=refnum<class "Data.lvclass"> refnum ("Data.lvclass")) -> ("Data out"=w1279:refnum<class "Data.lvclass">)  [unwired: 9 in]
                }
                frame 210 {
                  # "DTYPE_EVENT"
                  n496 = call-dynamic "Get Object Pointer.vi"("Data in"=w1285) -> ("Object Pointer"=w1281:i64)  [unwired: 8 in, 2 out]
                  n497 = call <vilib>:"Shared Set Object Pointer.vi"("Object Pointer"=w1281, "Data in"=refnum<class "Data.lvclass"> refnum ("Data.lvclass")) -> ("Data out"=w1284:refnum<class "Data.lvclass">)  [unwired: 9 in]
                }
                frame 211 {
                  # "DTYPE_WITH_UNITS"
                  n498 = call-dynamic "Get Object Pointer.vi"("Data in"=w1290) -> ("Object Pointer"=w1286:i64)  [unwired: 8 in, 2 out]
                  n499 = call <vilib>:"Shared Set Object Pointer.vi"("Object Pointer"=w1286, "Data in"=refnum<class "Data.lvclass"> refnum ("Data.lvclass")) -> ("Data out"=w1289:refnum<class "Data.lvclass">)  [unwired: 9 in]
                }
                frame 212 {
                  # "DTYPE_CALL"
                  n500 = call-dynamic "Get Object Pointer.vi"("Data in"=w1295) -> ("Object Pointer"=w1291:i64)  [unwired: 8 in, 2 out]
                  n501 = call <vilib>:"Shared Set Object Pointer.vi"("Object Pointer"=w1291, "Data in"=refnum<class "Data.lvclass"> refnum ("Data.lvclass")) -> ("Data out"=w1294:refnum<class "Data.lvclass">)  [unwired: 9 in]
                }
                frame 213 {
                  # "DTYPE_WITH_ERROR"
                  n502 = call-dynamic "Get Object Pointer.vi"("Data in"=w1300) -> ("Object Pointer"=w1296:i64)  [unwired: 8 in, 2 out]
                  n503 = call <vilib>:"Shared Set Object Pointer.vi"("Object Pointer"=w1296, "Data in"=refnum<class "Data.lvclass"> refnum ("Data.lvclass")) -> ("Data out"=w1299:refnum<class "Data.lvclass">)  [unwired: 9 in]
                }
                frame 214 {
                  # "DTYPE_LIST"
                  n504 = call-dynamic "Get Object Pointer.vi"("Data in"=w1305) -> ("Object Pointer"=w1301:i64)  [unwired: 8 in, 2 out]
                  n505 = call <vilib>:"Shared Set Object Pointer.vi"("Object Pointer"=w1301, "Data in"=refnum<class "Data.lvclass"> refnum ("Data.lvclass")) -> ("Data out"=w1304:refnum<class "Data.lvclass">)  [unwired: 9 in]
                }
                frame 215 {
                  # "DTYPE_TUPLE"
                  n506 = call-dynamic "Get Object Pointer.vi"("Data in"=w1310) -> ("Object Pointer"=w1306:i64)  [unwired: 8 in, 2 out]
                  n507 = call <vilib>:"Shared Set Object Pointer.vi"("Object Pointer"=w1306, "Data in"=refnum<class "Data.lvclass"> refnum ("Data.lvclass")) -> ("Data out"=w1309:refnum<class "Data.lvclass">)  [unwired: 9 in]
                }
                frame 216 {
                  # "DTYPE_DICTIONARY"
                  n508 = call-dynamic "Get Object Pointer.vi"("Data in"=w1315) -> ("Object Pointer"=w1311:i64)  [unwired: 8 in, 2 out]
                  n509 = call <vilib>:"Shared Set Object Pointer.vi"("Object Pointer"=w1311, "Data in"=refnum<class "Data.lvclass"> refnum ("Data.lvclass")) -> ("Data out"=w1314:refnum<class "Data.lvclass">)  [unwired: 9 in]
                }
              }
            }
          }
        }
      }
    }
    frame Error {
    }
  }
  "error out" <- w5
  "Data out" <- w3
